vi "GUI.Config Test.vi"(11 "Path Config file":path=path "C:/Trabajo/Test Asic Javi_2021/CONFIG/configuracion_produccion+10mV_CTAV2022A.test") -> (3 "Path out":path)   [LabVIEW 2019]
uses:
  test.test de configuracion gui.ctl
  Test.ctl
  TEST.TEST CONFIG HW.ctl
  Rigol DP832/DP832_Control Channels.ctl
  TEST.TEST CONFIG TEST MATRIZ.ctl
  TEST.TEST CONFIG TEST.ctl
  TEST.TEST RESULT.ctl
  test_result fvasic.ctl
  TEST.TEST EXECUTION TEST.ctl
  TEST.TEST CONFIG VGA.ctl
  TEST.TEST TEST INFO.ctl
  TEST.TEST INFO PC.ctl
  GenPulse_configurar.ctl
  machine estate configs.ctl
  Test_Conjunto Folder/Rigol DP832/DP832_Control Behavior.ctl
panel:
  out "CONFIG GEN temp":T1[](array[typedef]) {"Vasic Theorical" min=1.0 max=1000000.0 step=1.0 format="%#_6pV"; "Frequency" min=0.001 max=333000000.0 step=1000.0 format="%#_6pHz"; "Leading Edge Time" min=1e-09 max=1.0 step=1e-10 format="%#_6ps"; "Trailing Edge Time" min=1e-09 max=1.0 step=1e-10 format="%#_6ps"; "Delay" min=0.0 max=1.0 step=1e-12 format="%#_6ps"; "Trigger Level Sync" items=["ECL", "TTL"]; "Trigger Sync Out" items=["AB"=3, "B"=2, "A"=1, "None"=0]; "Load" min=1.0 max=1000000.0 step=1.0 format="%#_6p"; "DC Offset" min=-10.0 max=10.0 step=0.1 format="%#_6pV"; "Amplitude" min=0.05 max=5.0 step=0.001 format="%#_6pV"; "Width Time" min=1.5e-09 max=1.0 step=1e-10 format="%#_6ps"; "Channel" items=["Channel1"=1, "Channel2"=2]}
  out "Primera llamada":bool=TRUE
  in  "CHECK vga":bool
  in  "VGA":T2={"VALUES VGA"=[], "TIME VGA"={"PULSE WIDTH"=0, "FRECUENCY PULSE"=0.0}} {"TIME VGA"."FRECUENCY PULSE" format="%.3p"; "TIME VGA"."PULSE WIDTH" format="%04x"}
  out "FT_Handle":u32
  in  "Test":T3={"Config HW"={"VISA Rigol DP832"="Rigol_DP832", "Config Rigol DP832"=[{"Channel"=0, "V Limit"=5.5, "I Limit"=0.5, "V Out"=5.0}, {"Channel"=1, "V Limit"=5.5, "I Limit"=0.8, "V Out"=5.0}, {"Channel"=2, "V Limit"=5.5, "I Limit"=0.2, "V Out"=0.0}], "CTA Test#"="CTA013 A", "FT_Handle"=0, "Espera acceso FT"=10, "VISA Tek MDO3104"="Rigol_DP832", "VISA Key 81160A"="Rigol_DP832"}, "Config Test"=[{"Vasic"=2.8, "Global Reset"=FALSE, "Test Register?"=FALSE, "Test ADC?"=FALSE, "Test ADC"={"Repeats ADC"=100, "Max Desviation"=0.1}, "Limits ADC"={"Low"=[1.9, 1.3, 0.65, 0.0, 1.6, 1.4, 1.4, 0.9, 2.1, 0.85, 1.9], "High"=[2.1, 1.5, 0.85, 0.1, 1.4, 1.2, 1.2, 0.7, 1.9, 0.65, 1.7]}, "Test Max PN Min NP?"=FALSE, "Limits Max PN Min NP"={"Max P Upper"=2.177000045776367, "Min P Upper"=1.474, "Max N Upper"=1.475, "Min N Upper"=0.818, "Max P Lower"=1.888, "Min P Lower "=1.321, "Max N Lower"=1.322, "Min N Lower"=0.73}, "Test Rate Scan?"=FALSE, "Vin Rate Scan"=[], "Limits Rate Scan"={"High"=[0.15, 0.242, 0.331, 0.425, 0.512, 0.6, 0.688, 0.774, 0.847, 0.91], "Low"=[0.021, 0.11, 0.189, 0.27, 0.347, 0.421, 0.487, 0.551, 0.601, 0.635]}, "Test Rate Scan Adders?"=FALSE, "Vin Rate Adders"=[], "Limits Rate Scan adders"={"High"=[], "Low"=[]}, "Test offset analog?"=FALSE, "Lim Offset Analog"={"Max Analog"=0.05, "Min Analog"=-0.05}, "Test offset digital?"=FALSE, "Lim offset Dig"={"Max Dig"=0.05}, "Vasic real f.a."=2.8, "IBIAS"=FALSE, "VALUE IBIAS"=63}, {"Vasic"=2.8, "Global Reset"=FALSE, "Test Register?"=FALSE, "Test ADC?"=FALSE, "Test ADC"={"Repeats ADC"=100, "Max Desviation"=0.1}, "Limits ADC"={"Low"=[1.9, 1.3, 0.65, 0.0, 1.6, 1.4, 1.4, 0.9, 2.1, 0.85, 1.9], "High"=[2.1, 1.5, 0.85, 0.1, 1.4, 1.2, 1.2, 0.7, 1.9, 0.65, 1.7]}, "Test Max PN Min NP?"=FALSE, "Limits Max PN Min NP"={"Max P Upper"=2.177000045776367, "Min P Upper"=1.474, "Max N Upper"=1.475, "Min N Upper"=0.818, "Max P Lower"=1.888, "Min P Lower "=1.321, "Max N Lower"=1.322, "Min N Lower"=0.73}, "Test Rate Scan?"=FALSE, "Vin Rate Scan"=[], "Limits Rate Scan"={"High"=[0.15, 0.242, 0.331, 0.425, 0.512, 0.6, 0.688, 0.774, 0.847, 0.91], "Low"=[0.021, 0.11, 0.189, 0.27, 0.347, 0.421, 0.487, 0.551, 0.601, 0.635]}, "Test Rate Scan Adders?"=FALSE, "Vin Rate Adders"=[], "Limits Rate Scan adders"={"High"=[], "Low"=[]}, "Test offset analog?"=FALSE, "Lim Offset Analog"={"Max Analog"=0.05, "Min Analog"=-0.05}, "Test offset digital?"=FALSE, "Lim offset Dig"={"Max Dig"=0.05}, "Vasic real f.a."=2.8, "IBIAS"=FALSE, "VALUE IBIAS"=63}, {"Vasic"=2.8, "Global Reset"=FALSE, "Test Register?"=FALSE, "Test ADC?"=FALSE, "Test ADC"={"Repeats ADC"=100, "Max Desviation"=0.1}, "Limits ADC"={"Low"=[1.9, 1.3, 0.65, 0.0, 1.6, 1.4, 1.4, 0.9, 2.1, 0.85, 1.9], "High"=[2.1, 1.5, 0.85, 0.1, 1.4, 1.2, 1.2, 0.7, 1.9, 0.65, 1.7]}, "Test Max PN Min NP?"=FALSE, "Limits Max PN Min NP"={"Max P Upper"=2.177000045776367, "Min P Upper"=1.474, "Max N Upper"=1.475, "Min N Upper"=0.818, "Max P Lower"=1.888, "Min P Lower "=1.321, "Max N Lower"=1.322, "Min N Lower"=0.73}, "Test Rate Scan?"=FALSE, "Vin Rate Scan"=[], "Limits Rate Scan"={"High"=[0.15, 0.242, 0.331, 0.425, 0.512, 0.6, 0.688, 0.774, 0.847, 0.91], "Low"=[0.021, 0.11, 0.189, 0.27, 0.347, 0.421, 0.487, 0.551, 0.601, 0.635]}, "Test Rate Scan Adders?"=FALSE, "Vin Rate Adders"=[], "Limits Rate Scan adders"={"High"=[], "Low"=[]}, "Test offset analog?"=FALSE, "Lim Offset Analog"={"Max Analog"=0.05, "Min Analog"=-0.05}, "Test offset digital?"=FALSE, "Lim offset Dig"={"Max Dig"=0.05}, "Vasic real f.a."=2.8, "IBIAS"=FALSE, "VALUE IBIAS"=63}, {"Vasic"=2.8, "Global Reset"=FALSE, "Test Register?"=FALSE, "Test ADC?"=FALSE, "Test ADC"={"Repeats ADC"=100, "Max Desviation"=0.1}, "Limits ADC"={"Low"=[1.9, 1.3, 0.65, 0.0, 1.6, 1.4, 1.4, 0.9, 2.1, 0.85, 1.9], "High"=[2.1, 1.5, 0.85, 0.1, 1.4, 1.2, 1.2, 0.7, 1.9, 0.65, 1.7]}, "Test Max PN Min NP?"=FALSE, "Limits Max PN Min NP"={"Max P Upper"=2.177000045776367, "Min P Upper"=1.474, "Max N Upper"=1.475, "Min N Upper"=0.818, "Max P Lower"=1.888, "Min P Lower "=1.321, "Max N Lower"=1.322, "Min N Lower"=0.73}, "Test Rate Scan?"=FALSE, "Vin Rate Scan"=[], "Limits Rate Scan"={"High"=[0.15, 0.242, 0.331, 0.425, 0.512, 0.6, 0.688, 0.774, 0.847, 0.91], "Low"=[0.021, 0.11, 0.189, 0.27, 0.347, 0.421, 0.487, 0.551, 0.601, 0.635]}, "Test Rate Scan Adders?"=FALSE, "Vin Rate Adders"=[], "Limits Rate Scan adders"={"High"=[], "Low"=[]}, "Test offset analog?"=FALSE, "Lim Offset Analog"={"Max Analog"=0.05, "Min Analog"=-0.05}, "Test offset digital?"=FALSE, "Lim offset Dig"={"Max Dig"=0.05}, "Vasic real f.a."=2.8, "IBIAS"=FALSE, "VALUE IBIAS"=63}], "Result"=[], "Execucion Test"={"Vasic Actual"=0}, "Config VGA"={"Theoretical Voltage"=[0.1, 0.2, 0.3, 0.4, 0.5, 0.6, 0.7, 0.8, 0.9, 1.0], "Real Voltage"=[0.10285, 0.20714, 0.29957, 0.40485, 0.49571, 0.60685, 0.69771, 0.80114, 0.89714, 0.99885], "Pulse Width"=57344, "Frecuency Pulse"=1000000.0, "VGA Gain"=[9, 16, 24, 34, 43, 52, 61, 72, 81, 93]}, "Test Info"={"Asic"="", "Operator"="", "Place"="", "Time start"=timestamp(0 s since 1904-01-01), "Time stop"=timestamp(0 s since 1904-01-01)}, "Info machine"={"SO"="", "SO Name"="", "SO Ver"="", "SO Build"="", "CPU"="", "APP"="", "APP YEAR"="", "APP ver"="", "APP User"="", "APP Serail"="", "MAC"=[], "PC NAME"=[], "PC IP"=[], "BIOS MANU"="", "BIOS NAME"="", "BIOS SERIAL"="", "BOARD MANU"="", "BOARD NAME"="", "BOARD SERIAL"="", "Driver Version"="", "Library Version"="", "FPGA Ver"=0, "ID CTA board"=0, "LAST BOOT"="", "LABVIEW Ver"=0}, "Partial Report"="", "CONFIG GEN"=[]} {"CONFIG GEN"."Vasic Theorical" min=1.0 max=1000000.0 step=1.0 format="%#_6pV"; "CONFIG GEN"."Frequency" min=0.001 max=333000000.0 step=1000.0 format="%#_6pHz"; "CONFIG GEN"."Leading Edge Time" min=1e-09 max=1.0 step=1e-10 format="%#_6ps"; "CONFIG GEN"."Trailing Edge Time" min=1e-09 max=1.0 step=1e-10 format="%#_6ps"; "CONFIG GEN"."Delay" min=0.0 max=1.0 step=1e-12 format="%#_6ps"; "CONFIG GEN"."Trigger Level Sync" items=["ECL", "TTL"]; "CONFIG GEN"."Trigger Sync Out" items=["AB"=3, "B"=2, "A"=1, "None"=0]; "CONFIG GEN"."Load" min=1.0 max=1000000.0 step=1.0 format="%#_6p"; "CONFIG GEN"."DC Offset" min=-10.0 max=10.0 step=0.1 format="%#_6pV"; "CONFIG GEN"."Amplitude" min=0.05 max=5.0 step=0.001 format="%#_6pV"; "CONFIG GEN"."Width Time" min=1.5e-09 max=1.0 step=1e-10 format="%#_6ps"; "CONFIG GEN"."Channel" items=["Channel1"=1, "Channel2"=2]; "Config VGA"."Theoretical Voltage" format="%1.4f"; "Config VGA"."VGA Gain" format="%02x"; "Config VGA"."Frecuency Pulse" format="%0_2p"; "Config VGA"."Pulse Width" format="%04x"; "Config VGA"."Real Voltage" format="%1.5f"; "Config Test"."VALUE IBIAS" max=63 step=1; "Config Test"."Vasic real f.a." min=2.8 max=3.8 step=0.01 format="%.2g"; "Config Test"."Limits Rate Scan adders"."Low" format="%1.3f"; "Config Test"."Limits Rate Scan adders"."High" format="%1.3f"; "Config Test"."Limits ADC"."High" format="%1.4f"; "Config Test"."Limits ADC"."Low" format="%1.3f"; "Config Test"."Lim offset Dig"."Max Dig" format="%.3g"; "Config Test"."Lim Offset Analog"."Min Analog" format="%.3g"; "Config Test"."Lim Offset Analog"."Max Analog" format="%.3g"; "Config Test"."Limits Rate Scan"."Low" format="%1.4f"; "Config Test"."Limits Rate Scan"."High" format="%1.3f"; "Config Test"."Limits Max PN Min NP"."Min P Upper" format="%.3g"; "Config Test"."Limits Max PN Min NP"."Min P Lower" format="%.3g"; "Config Test"."Limits Max PN Min NP"."Max N Lower" format="%.3g"; "Config Test"."Limits Max PN Min NP"."Max N Upper" format="%.3g"; "Config Test"."Limits Max PN Min NP"."Min N Lower" format="%.3g"; "Config Test"."Limits Max PN Min NP"."Min N Upper" format="%.3g"; "Config Test"."Limits Max PN Min NP"."Max P Upper" format="%.3g"; "Config Test"."Limits Max PN Min NP"."Max P Lower" format="%.3g"; "Config Test"."Vasic" min=2.8 max=3.8 step=0.01 format="%.2g"; "Config HW"."Config Rigol DP832"."Channel" items=["+30V Channel 1", "+30V Channel 2", "+5V Channel 3"]; "Config HW"."Config Rigol DP832"."V Limit" format="%.1g"; "Config HW"."Config Rigol DP832"."I Limit" format="%.1g"; "Config HW"."Config Rigol DP832"."V Out" format="%.1g"; "Result"."Test Registros"."Read W/R" format="%04x"; "Result"."Test Registros"."Pattern W/R" format="%04x"; "Result"."Test Registros"."Read Default" format="%04x"; "Result"."Test Registros"."Pattern Default" format="%04x"}
  in  "visualize":enum32{"Page 1", "Page 2"}(tab)
  in  "Change value Gen":bool
  in  "VISA Oscilloscope Tek MDO3104":refnum<visa-resource-name>
  in  "VISA Generator Key 81160A":refnum<visa-resource-name>
  in  "Elemensts":i32(listbox)=-1
  in  "vga test":T14={"FRECUENCY PULSE"=-0.05, "PULSE WIDTH"=0, "CODE GAIN TEST"=0} {"CODE GAIN TEST" max=127 step=1; "PULSE WIDTH" format="%04x"; "FRECUENCY PULSE" format="%.3p"}
  in  "CTA Board":string(combo)
  in  "CHECK cta":bool
  in  "CHECK POWER":bool
  in  "Config Rigol DP832":T15(array[cluster]) {"Channel" items=["+30V Channel 1", "+30V Channel 2", "+5V Channel 3"]; "V Limit" min=0.0 max=6.0 step=0.1 format="%.1g"; "I Limit" min=0.0 max=1.0 step=0.1 format="%.1g"; "V Out" min=0.0 max=6.0 step=0.01 format="%.2g"}
  in  "copy to new":bool
  in  "new":bool
  in  "delete":bool
  in  "Valores":T16[](array[typedef]) {"VALUE IBIAS" max=63 step=1; "V SUPPLY ASIC REAL" min=2.5 max=3.6 step=0.01 format="%.2g"; "VOLTAGE SUPPLY ASIC" min=2.5 max=3.5 step=0.05 format="%.2g"; "LIMITS OFFSET DIGITAL"."MAXIMUM" format="%.3g"; "LIMITS OFFSET ANALOG"."MINIMUM" format="%.3g"; "LIMITS OFFSET ANALOG"."MAXIMUM" format="%.3g"; "SETUP ADC"."MAX DESVIATION ADC" format="%.3g"}
  in  "default":bool
  in  "Load config":bool
  in  "save config":bool
  in  "QUIT":bool
  in  "VISA Rigol DP832":refnum<visa-resource-name>
  out "Values Gen":string[][](table)
  out "Cambios":bool
  # "Modo 2\nModo 3\nModo 4\nModo 2\nModo 3\nModo 4"
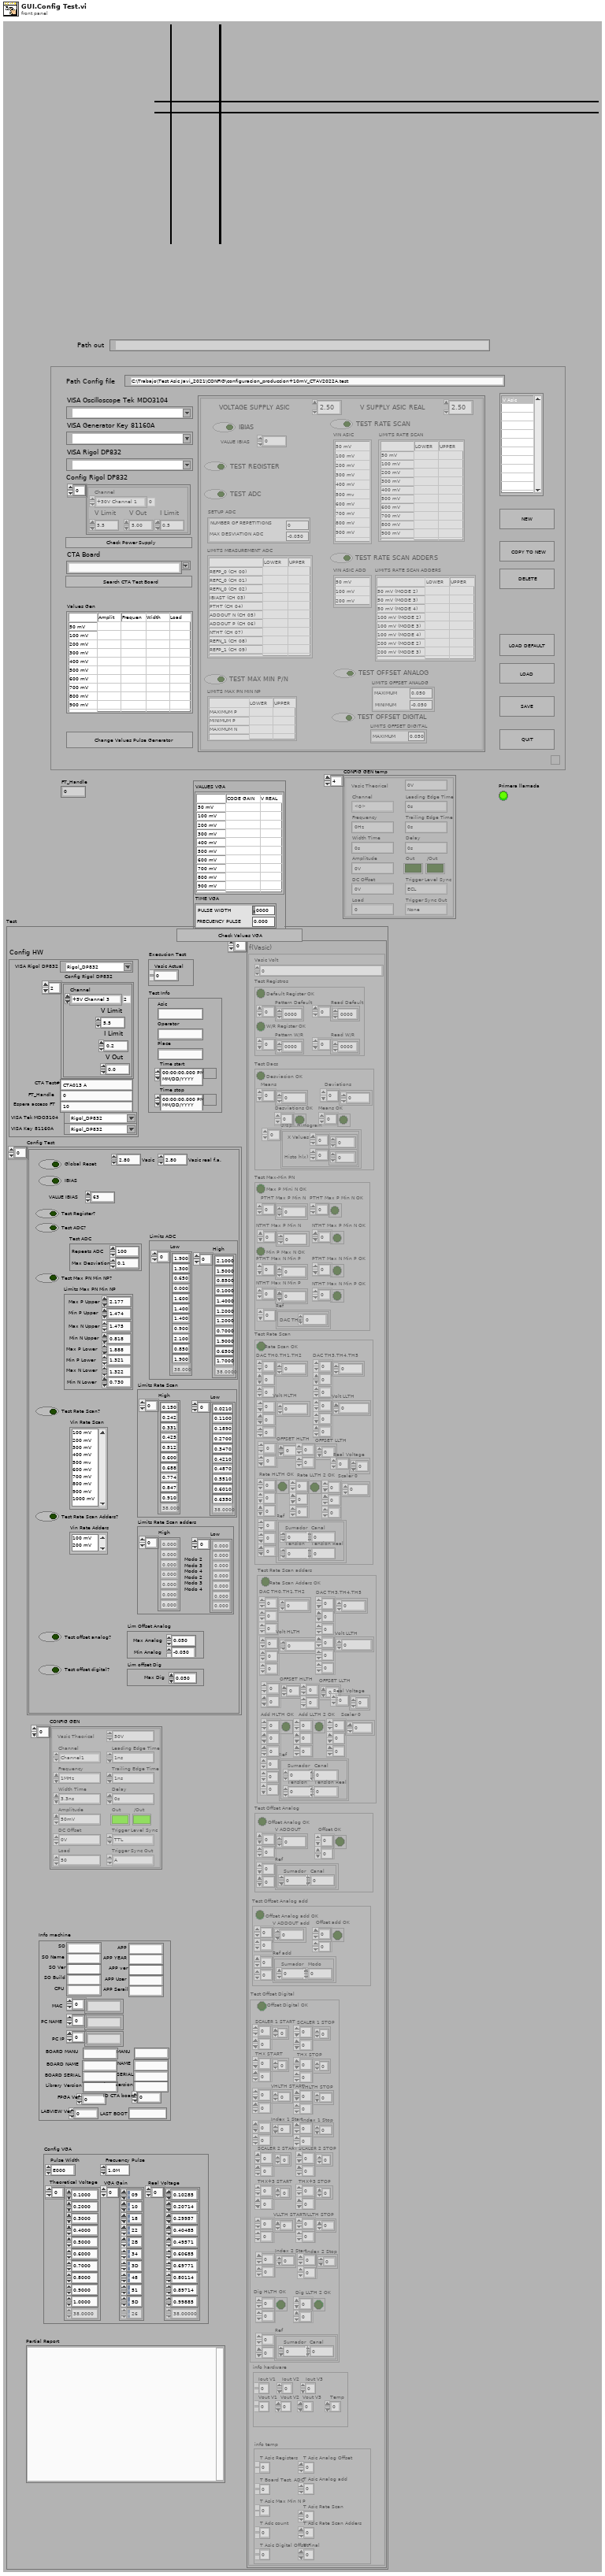
[diagram p1: front panel]
types:
  T1 = typedef "GenPulse_configurar.ctl" = cluster{"Channel":u16, "Frequency":dbl, "Width Time":dbl, "Amplitude":dbl, "DC Offset":dbl, "Load":dbl, "Leading Edge Time":dbl, "Trailing Edge Time":dbl, "Delay":dbl, "Out":bool, "/Out":bool, "Trigger Level Sync":u16, "Trigger Sync Out":u16, "Vasic Theorical":dbl}
  T2 = cluster{"VALUES VGA":string[][], "TIME VGA":cluster{"PULSE WIDTH":u16, "FRECUENCY PULSE":dbl}}
  T3 = typedef "Test.ctl" = cluster{"Config HW":T4, "Config Test":T6, "Result":T8, "Execucion Test":T10, "Config VGA":T11, "Test Info":T12, "Info machine":T13, "Partial Report":string, "CONFIG GEN":T1[]}
  T4 = typedef "TEST.TEST CONFIG HW.ctl" = cluster{"VISA Rigol DP832":refnum<visa-resource-name>, "Config Rigol DP832":cluster{"Channel":T5, "V Limit":dbl, "I Limit":dbl, "V Out":dbl}[], "CTA Test#":string, "FT_Handle":u32, "Espera acceso FT":u32, "VISA Tek MDO3104":refnum<visa-resource-name>, "VISA Key 81160A":refnum<visa-resource-name>}
  T5 = typedef "DP832_Control Channels.ctl" = i32
  T6 = typedef "TEST.TEST CONFIG TEST MATRIZ.ctl" = T7[]
  T7 = typedef "TEST.TEST CONFIG TEST.ctl" = cluster{"Vasic":dbl, "Global Reset":bool, "Test Register?":bool, "Test ADC?":bool, "Test ADC":cluster{"Repeats ADC":i32, "Max Desviation":dbl}, "Limits ADC":cluster{"Low":dbl[], "High":dbl[]}, "Test Max PN Min NP?":bool, "Limits Max PN Min NP":cluster{"Max P Upper":dbl, "Min P Upper":dbl, "Max N Upper":dbl, "Min N Upper":dbl, "Max P Lower":dbl, "Min P Lower ":dbl, "Max N Lower":dbl, "Min N Lower":dbl}, "Test Rate Scan?":bool, "Vin Rate Scan":i32[], "Limits Rate Scan":cluster{"High":dbl[], "Low":dbl[]}, "Test Rate Scan Adders?":bool, "Vin Rate Adders":i32[], "Limits Rate Scan adders":cluster{"High":dbl[], "Low":dbl[]}, "Test offset analog?":bool, "Lim Offset Analog":cluster{"Max Analog":dbl, "Min Analog":dbl}, "Test offset digital?":bool, "Lim offset Dig":cluster{"Max Dig":dbl}, "Vasic real f.a.":dbl, "IBIAS":bool, "VALUE IBIAS":u8}
  T8 = typedef "TEST.TEST RESULT.ctl" = T9[]
  T9 = typedef "test_result fvasic.ctl" = cluster{"Vasic Volt":i32, "Test Registros":cluster{"Default Register OK":bool, "Pattern Default":u16[], "Read Default":u16[], "W/R Register OK":bool, "Pattern W/R":u16[], "Read W/R":u16[]}, "Test Dacs":cluster{"Desviacion OK":bool, "Means":dbl[], "Deviations":dbl[], "Desviations OK":bool[], "Means OK":bool[], "Graph Histogram":cluster{"X Values":dbl[], "Histo h(x)":i32[]}[]}, "Test Max-Min PN":cluster{"Max P Mini N OK":bool, "PTHT Max P Min N":dbl[], "PTHT Max P Min N OK":bool[], "NTHT Max P Min N":dbl[], "NTHT Max P Min N OK":bool[], "Min P Max N OK":bool, "PTHT Max N Min P":dbl[], "PTHT Max N Min P OK":bool[], "NTHT Max N Min P":dbl[], "NTHT Max N Min P OK":bool[], "Ref":cluster{"DAC THx":u8}[]}, "Test Rate Scan":cluster{"Rate Scan OK":bool, "DAC TH0,TH1,TH2":u16[][][], "Volt HLTH":dbl[][][], "Rate HLTH OK":bool[][][], "DAC TH3,TH4,TH5":u16[][][], "Volt LLTH":dbl[][][], "Rate LLTH 2 OK":bool[][][], "Scaler 0":u16[][][], "Ref":cluster{"Sumador":u8, "Canal":u8, "Tension":u8, "Tension Real":dbl}[][][], "OFFSET HLTH":dbl[][], "OFFSET LLTH":dbl[][], "Real Voltage":dbl[]}, "Test Rate Scan adders":cluster{"Rate Scan Adders OK":bool, "DAC TH0,TH1,TH2":u16[][][], "Volt HLTH":dbl[][][], "Add HLTH OK":bool[][][], "DAC TH3,TH4,TH5":u16[][][], "Volt LLTH":dbl[][][], "Add LLTH 2 OK":bool[][][], "Scaler 0":u16[][][], "Ref":cluster{"Sumador":u8, "Canal":u8, "Tension":u8, "Tension Real":dbl}[][][], "OFFSET HLTH":dbl[][], "OFFSET LLTH":dbl[][], "Real Voltage":dbl[]}, "Test Offset Analog":cluster{"Offset Analog OK":bool, "V ADDOUT":dbl[][], "Offset OK":bool[][], "Ref":cluster{"Sumador":u8, "Canal":u8}[][]}, "Test Offset Digital":cluster{"Offset Digital OK":bool, "SCALER 1 START":u16[][], "SCALER 1 STOP":u16[][], "THX START":u16[][], "THX STOP":u16[][], "VHLTH START":dbl[][], "VHLTH STOP":dbl[][], "Index 1 Start":i32[][], "index 1 Stop":i32[][], "SCALER 2 START":u16[][], "SCALER 2 STOP":u16[][], "THX+3 START":u16[][], "THX+3 STOP":u16[][], "VLLTH START":dbl[][], "VLLTH STOP":dbl[][], "Index 2 Start":i32[][], "index 2 Stop":i32[][], "Dig HLTH OK":bool[][], "Dig LLTH 2 OK":bool[][], "Ref":cluster{"Sumador":u8, "Canal":u8}[][]}, "info hardware":cluster{"Iout V1":dbl, "Iout V2":dbl, "Iout V3":dbl, "Vout V1":dbl, "Vout V2":dbl, "Vout V3":dbl, "Temp":dbl}, "Test Offset Analog add":cluster{"Offset Analog add OK":bool, "V ADDOUT add":dbl[][], "Offset add OK":bool[][], "Ref add":cluster{"Sumador":u8, "Modo":u8}[][]}, "info temp":cluster{"T Asic Registers":dbl, "T Board Test. ADC":dbl, "T Asic Max Min N P":dbl, "T Adc count":dbl, "T Asic Digital Offset":dbl, "T Asic Analog Offset":dbl, "T Asic Analog add":dbl, "T Asic Rate Scan":dbl, "T Asic Rate Scan Adders":dbl, "T Final":dbl}}
  T10 = typedef "TEST.TEST EXECUTION TEST.ctl" = cluster{"Vasic Actual":i32}
  T11 = typedef "TEST.TEST CONFIG VGA.ctl" = cluster{"Theoretical Voltage":dbl[], "Real Voltage":dbl[], "Pulse Width":u16, "Frecuency Pulse":dbl, "VGA Gain":u8[]}
  T12 = typedef "TEST.TEST TEST INFO.ctl" = cluster{"Asic":string, "Operator":string, "Place":string, "Time start":timestamp, "Time stop":timestamp}
  T13 = typedef "TEST.TEST INFO PC.ctl" = cluster{"SO":string, "SO Name":string, "SO Ver":string, "SO Build":string, "CPU":string, "APP":string, "APP YEAR":string, "APP ver":string, "APP User":string, "APP Serail":string, "MAC":string[], "PC NAME":string[], "PC IP":string[], "BIOS MANU":string, "BIOS NAME":string, "BIOS SERIAL":string, "BOARD MANU":string, "BOARD NAME":string, "BOARD SERIAL":string, "Driver Version":string, "Library Version":string, "FPGA Ver":u8, "ID CTA board":u64, "LAST BOOT":string, "LABVIEW Ver":u32}
  T14 = cluster{"FRECUENCY PULSE":dbl, "PULSE WIDTH":u16, "CODE GAIN TEST":u8}
  T15 = cluster{"Channel":T5, "V Limit":dbl, "I Limit":dbl, "V Out":dbl}[]
  T16 = typedef "test.test de configuracion gui.ctl" = cluster{"VOLTAGE SUPPLY ASIC":dbl, "GLOBAL RESET":bool, "TEST REGISTER":bool, "TEST ADC":bool, "SETUP ADC":cluster{"NUMBER OF REPETITIONS":i32, "MAX DESVIATION ADC":dbl}, "LIMITS MEASUREMENT ADC":string[][], "TEST MAX MIN P/N":bool, "LIMITS MAX PN MIN NP":string[][], "TEST RATE SCAN":bool, "VIN ASIC":i32[], "LIMITS RATE SCAN":string[][], "TEST RATE SCAN ADDERS":bool, "VIN ASIC ADD":i32[], "LIMITS RATE SCAN ADDERS":string[][], "TEST OFFSET ANALOG":bool, "LIMITS OFFSET ANALOG":cluster{"MAXIMUM":dbl, "MINIMUM":dbl}, "TEST OFFSET DIGITAL":bool, "LIMITS OFFSET DIGITAL":cluster{"MAXIMUM":dbl}, "V SUPPLY ASIC REAL":dbl, "VALUE IBIAS":u8, "IBIAS":bool}
  T17 = typedef "machine estate configs.ctl" = enum16{"Default values", "Init", "load init file", "wait", "Load File", "Refresh", "quit", "Save File", "Save In Config", "Valores>Test", "Test>View", "quit save"}
  T18 = cluster{"Config HW":T4, "Config Test":T6, "Config VGA":T11, "CONFIG GEN":T1[]}
  T19 = enum8{"Enabled", "Disabled", "Disabled and Grayed Out"}
  T20 = cluster{"Left Button Key Shortcut":cluster{"Control":bool, "Shift":bool, "Key":string}, "Center Button Key Shortcut":cluster{"Control":bool, "Shift":bool, "Key":string}, "Right Button Key Shortcut":cluster{"Control":bool, "Shift":bool, "Key":string}}
  T21 = cluster{"CTA Test#":string, "CTA Test#":string}[]
  T22 = typedef "DP832_Control Behavior.ctl" = u16
  T23 = cluster{"Device Index":u32, "FT_FLAGS_OPENED":bool, "FT_FLAGS_HISPEED":bool, "Type":u32, "VID":u32, "PID":u32, "LocID":i32, "Serial Number":string, "Description":string, "FT_Handle":u32}[]
  T24 = cluster{"Device Index":u32, "FT_FLAGS_OPENED":bool, "FT_FLAGS_HISPEED":bool, "Type":u32, "VID":u32, "PID":u32, "LocID":i32, "Serial Number":string, "Description":string, "FT_Handle":u32}
  T25 = cluster{"Serial Number":string, "Serial Number":string}
  T26 = cluster{"Vsupply asic":dbl, "Global Reset":bool, "Test Register??":bool, "Test ADC??":bool, "Test ADC set":cluster{"Repeats ADC":i32, "Max Desviation":dbl}, "High ADC means":dbl[], "Low ADC means":dbl[], "Test MAX/MIN??":bool, "Limits Max PN Min NP":cluster{"Max P Lower":dbl, "Min P Lower ":dbl, "Max N Lower":dbl, "Min N Lower":dbl, "Max P Upper":dbl, "Min P Upper":dbl, "Min N Upper":dbl, "Max N Upper":dbl}, "Test rate scan":bool, "Vin Rate Scan":i32[], "High rate scan":dbl[], "Low rate scan":dbl[], "Test rate scan adders??":bool, "Vin Rate Adders":i32[], "High rate scan add":dbl[], "Low rate scan add":dbl[], "Test offset analog??":bool, "Lim Offset Analog":cluster{"Max Analog":dbl, "Min Analog":dbl}, "Test offset digital??":bool, "Lim offset Dig":cluster{"Max Dig":dbl}, "Vsupply asic real":dbl, "IBIAS":bool, "VALUE IBIAS":u8}[]
  T27 = cluster{"Vsupply asic":dbl, "Global Reset":bool, "Test Register??":bool, "Test ADC??":bool, "Test ADC set":cluster{"Repeats ADC":i32, "Max Desviation":dbl}, "High ADC means":dbl[], "Low ADC means":dbl[], "Test MAX/MIN??":bool, "Limits Max PN Min NP":cluster{"Max P Lower":dbl, "Min P Lower ":dbl, "Max N Lower":dbl, "Min N Lower":dbl, "Max P Upper":dbl, "Min P Upper":dbl, "Min N Upper":dbl, "Max N Upper":dbl}, "Test rate scan":bool, "Vin Rate Scan":i32[], "High rate scan":dbl[], "Low rate scan":dbl[], "Test rate scan adders??":bool, "Vin Rate Adders":i32[], "High rate scan add":dbl[], "Low rate scan add":dbl[], "Test offset analog??":bool, "Lim Offset Analog":cluster{"Max Analog":dbl, "Min Analog":dbl}, "Test offset digital??":bool, "Lim offset Dig":cluster{"Max Dig":dbl}, "Vsupply asic real":dbl, "IBIAS":bool, "VALUE IBIAS":u8}
  T28 = enum16{"Left Button", "Center Button", "Right Button", "Window Close"}
  T29 = cluster{"VISA Rigol DP832":refnum<visa-resource-name>, "CTA Test#":string, "VISA Tek MDO3104":refnum<visa-resource-name>, "VISA Key 81160a":refnum<visa-resource-name>}
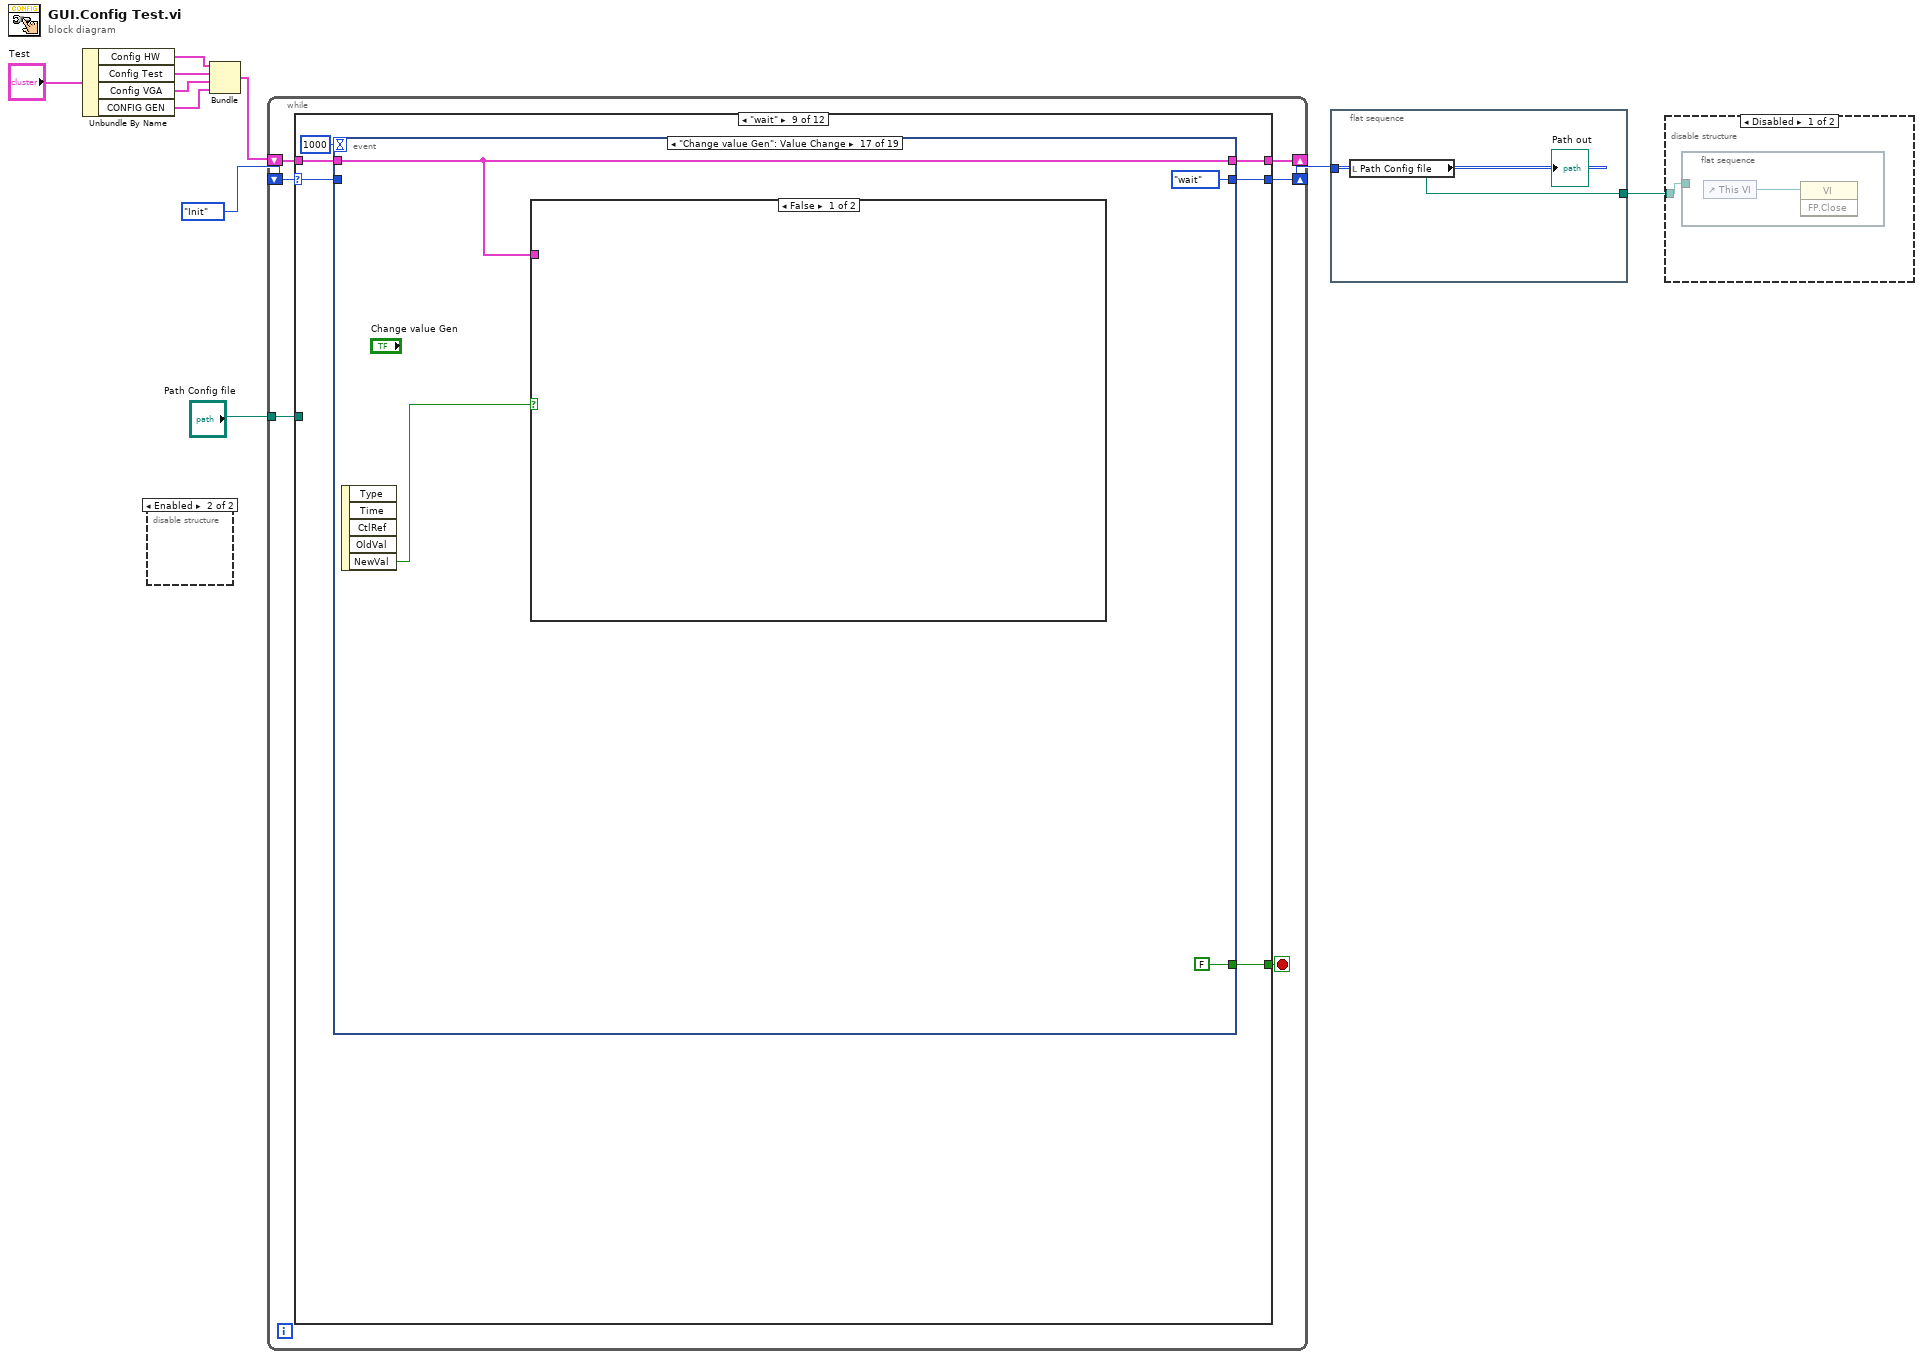
[diagram p0: block diagram]
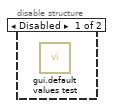
[diagram p3: hidden frame]
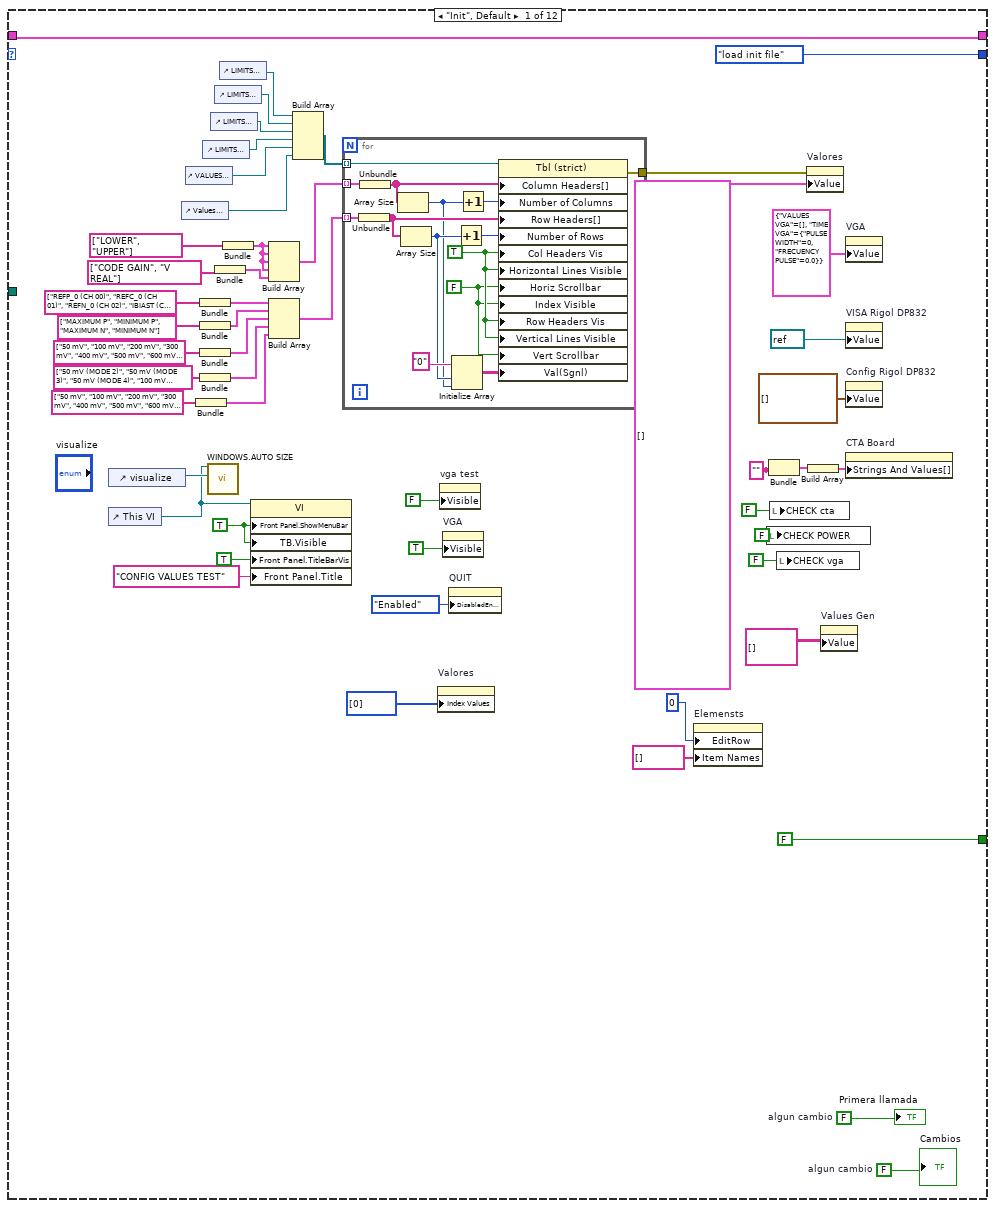
[diagram p4: hidden frame]
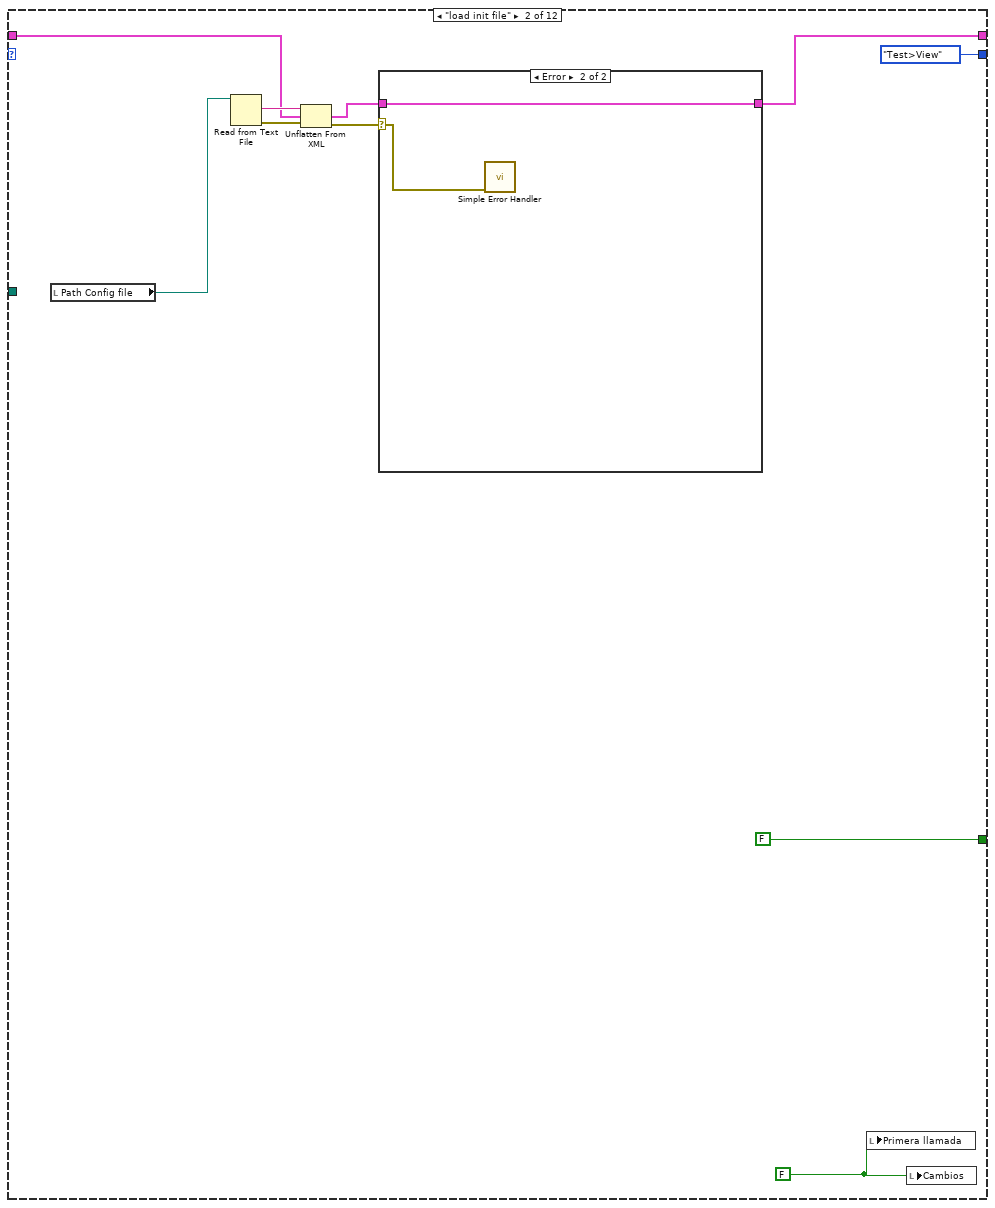
[diagram p5: hidden frame]
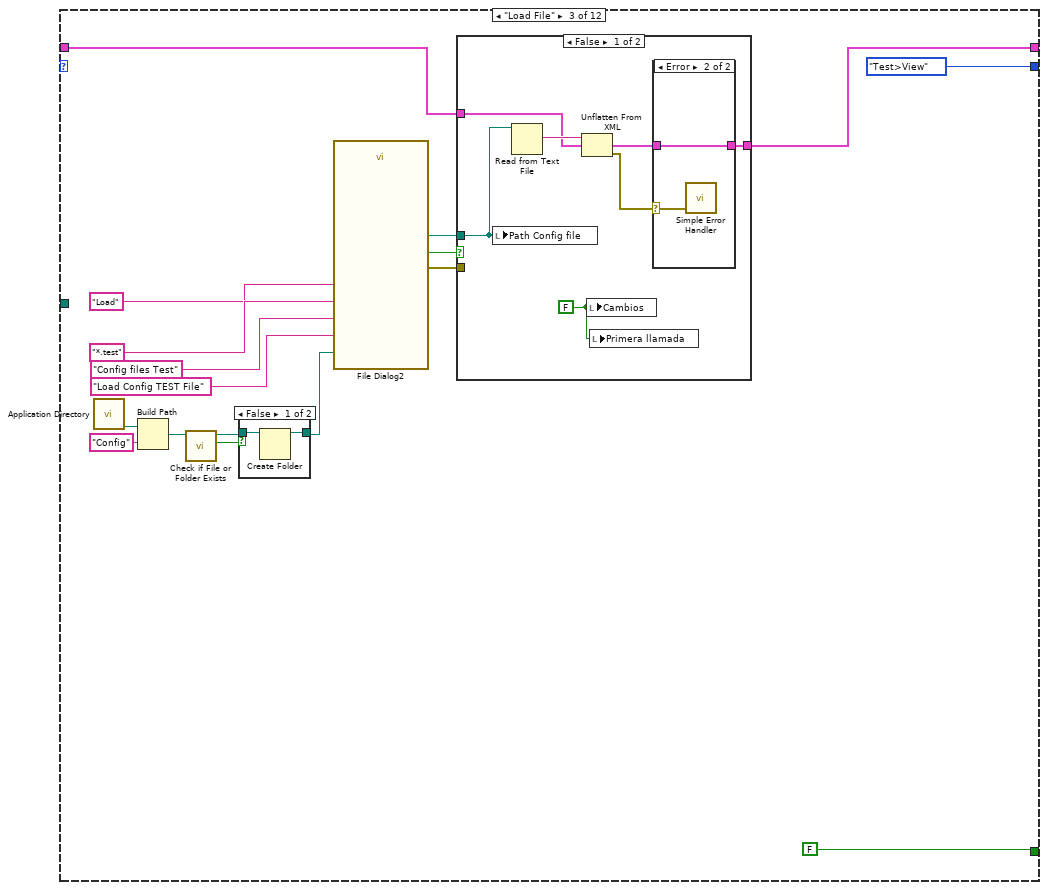
[diagram p7: hidden frame]
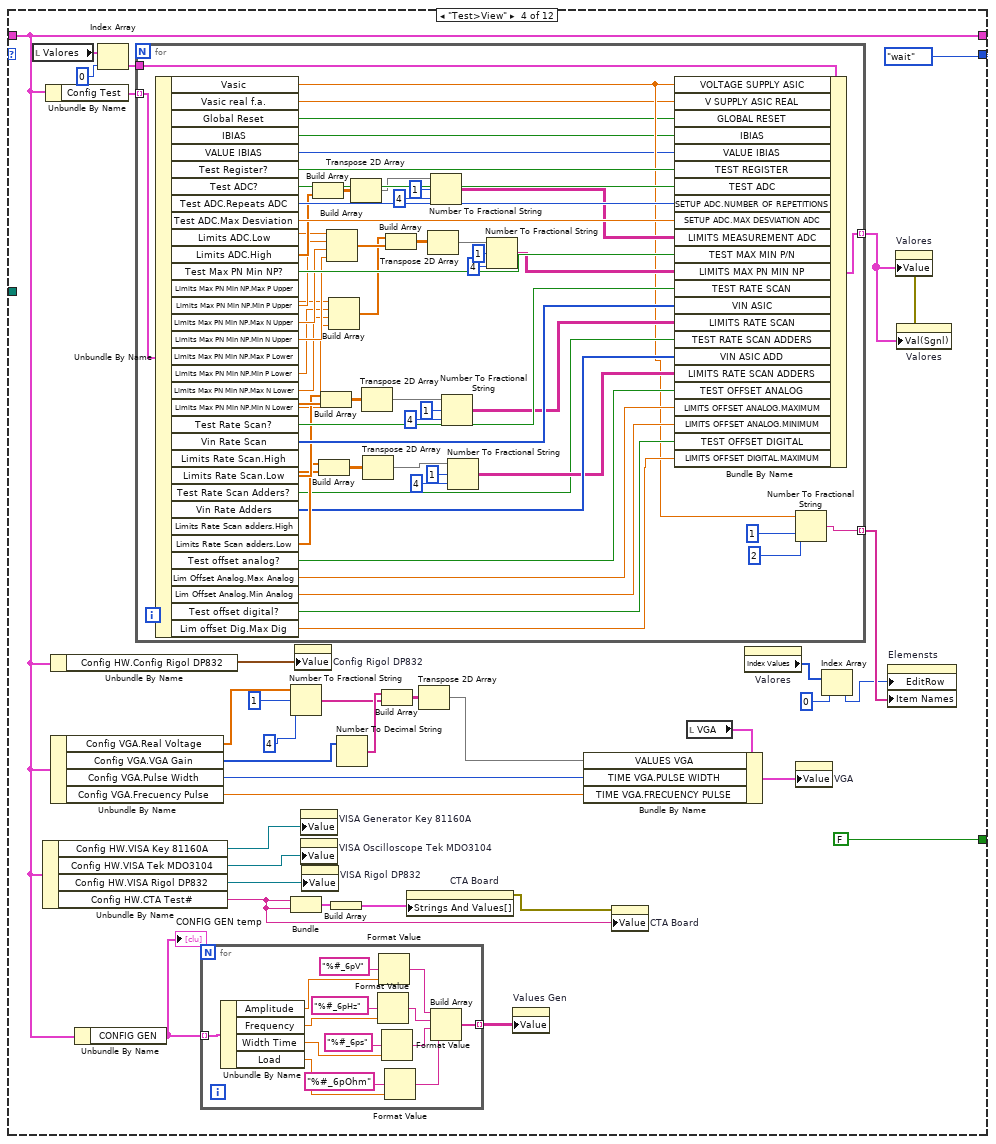
[diagram p11: hidden frame]
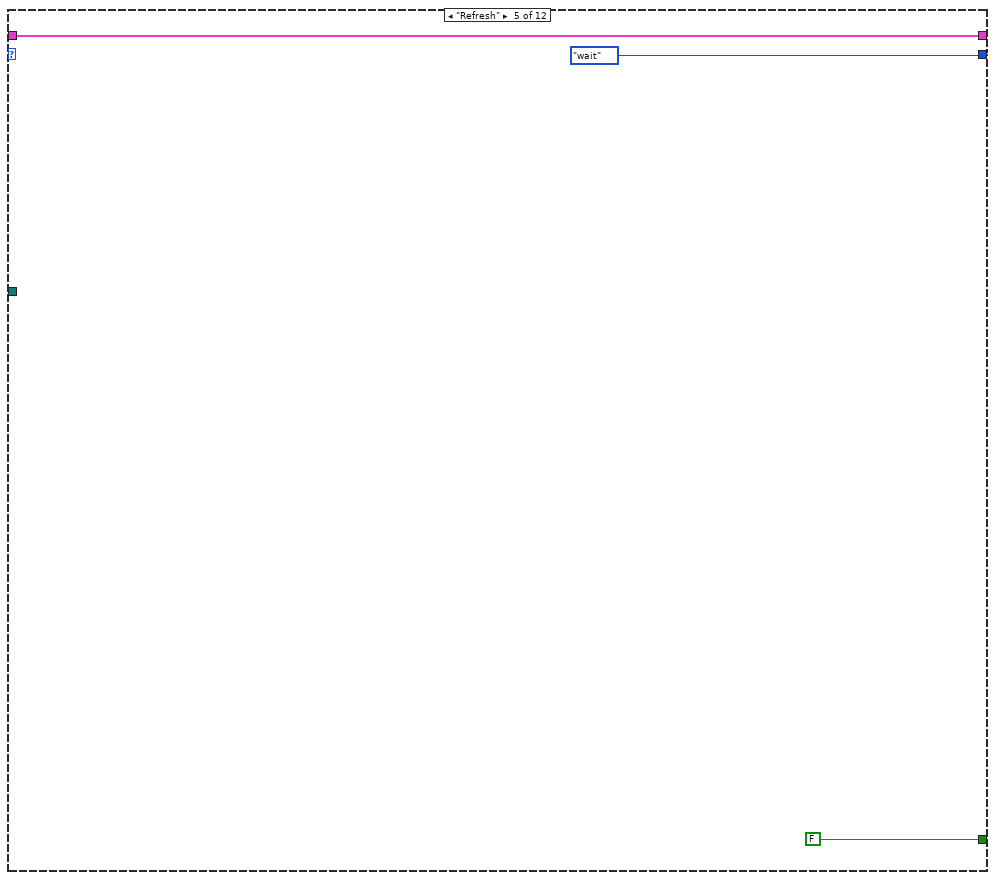
[diagram p12: hidden frame]
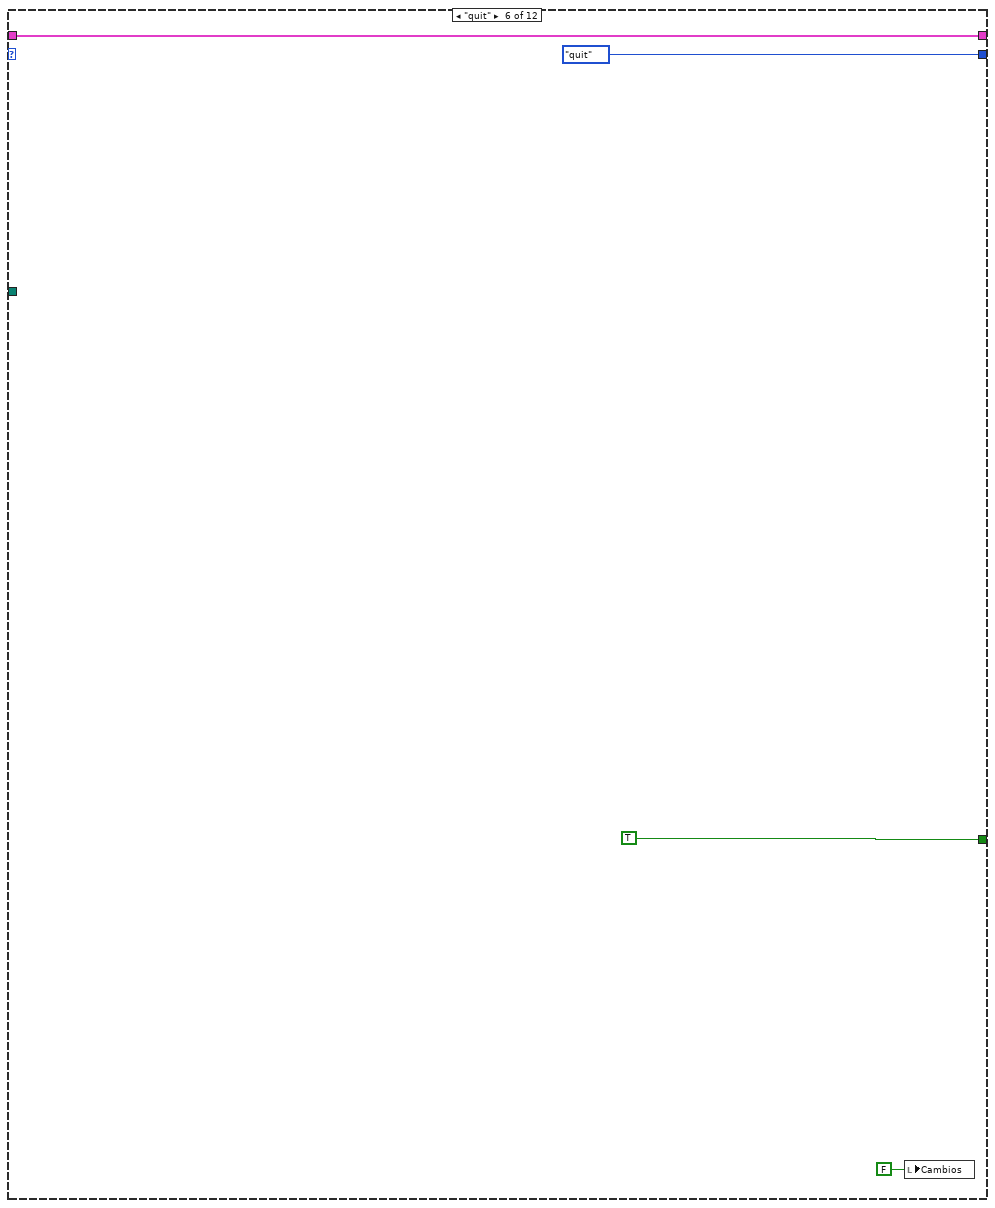
[diagram p13: hidden frame]
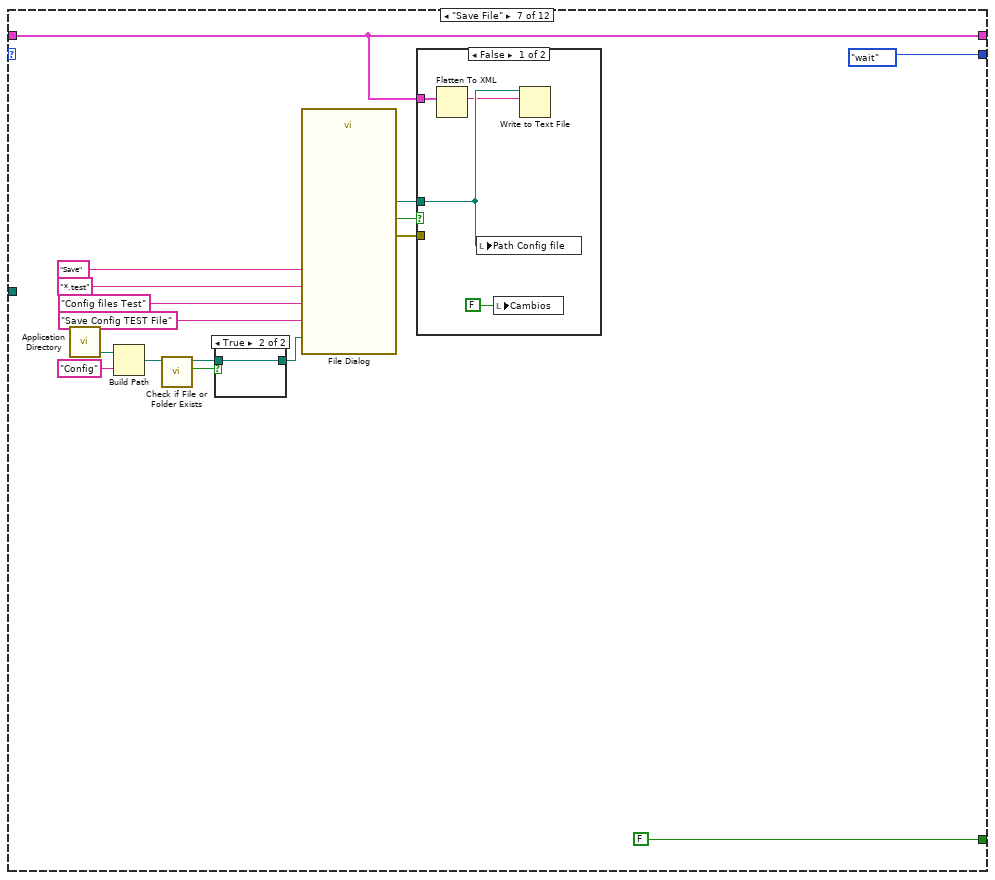
[diagram p14: hidden frame]
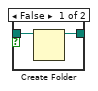
[diagram p16: hidden frame]
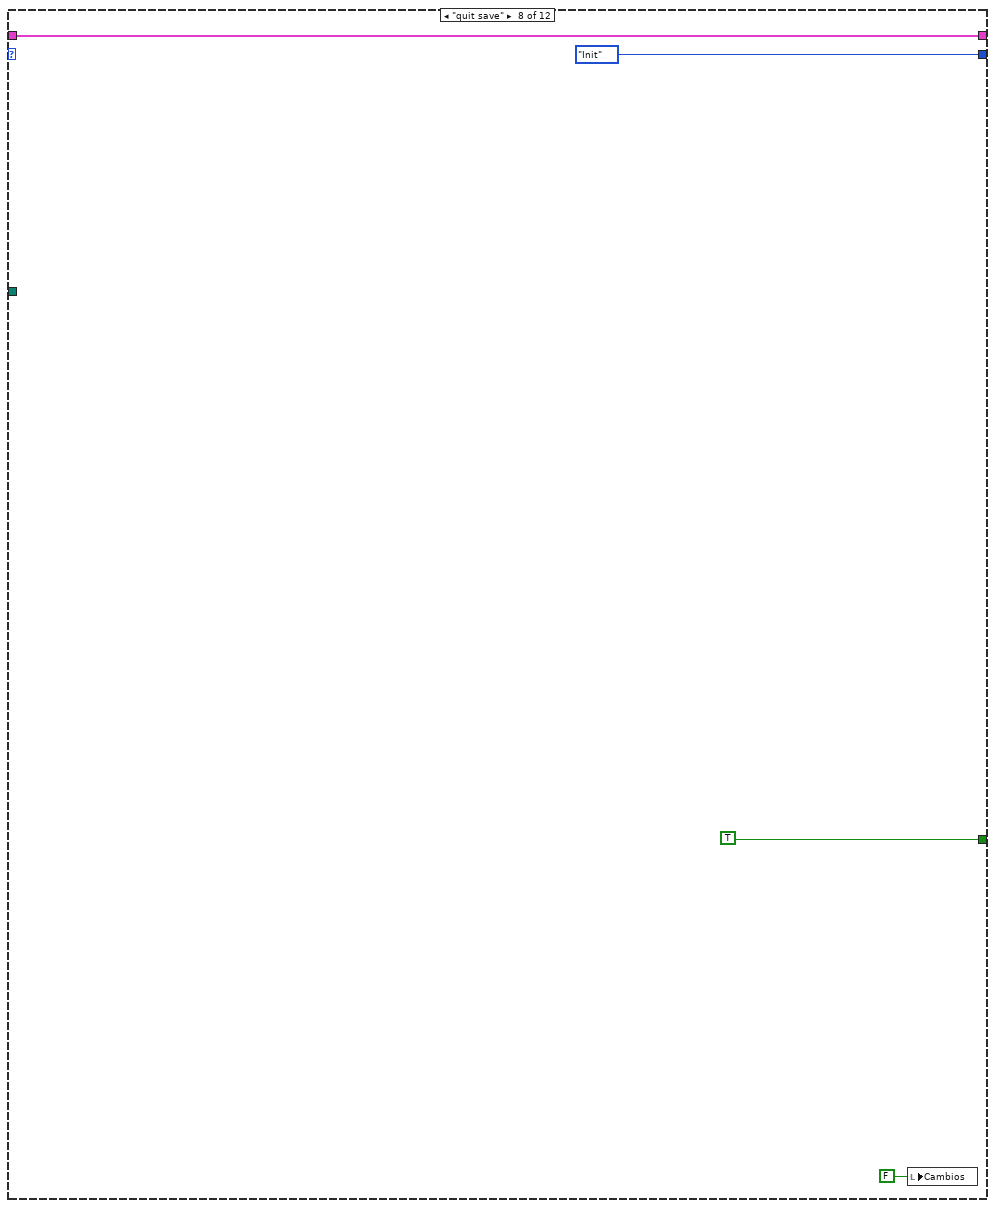
[diagram p17: hidden frame]
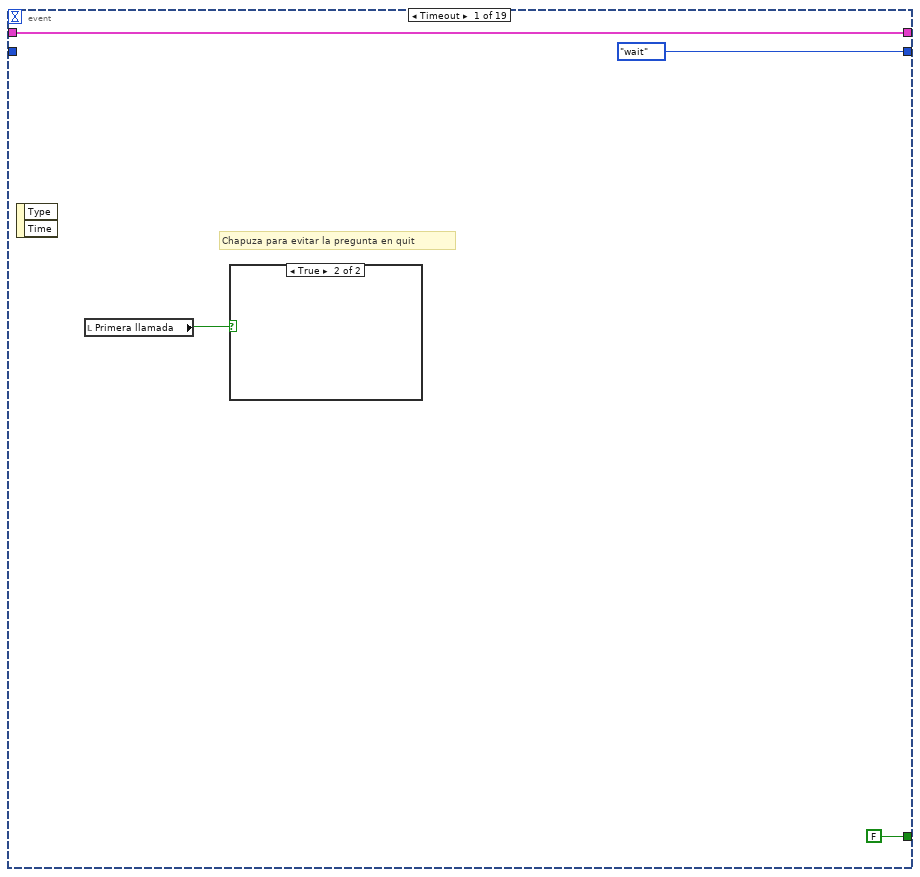
[diagram p18: hidden frame]
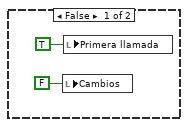
[diagram p19: hidden frame]
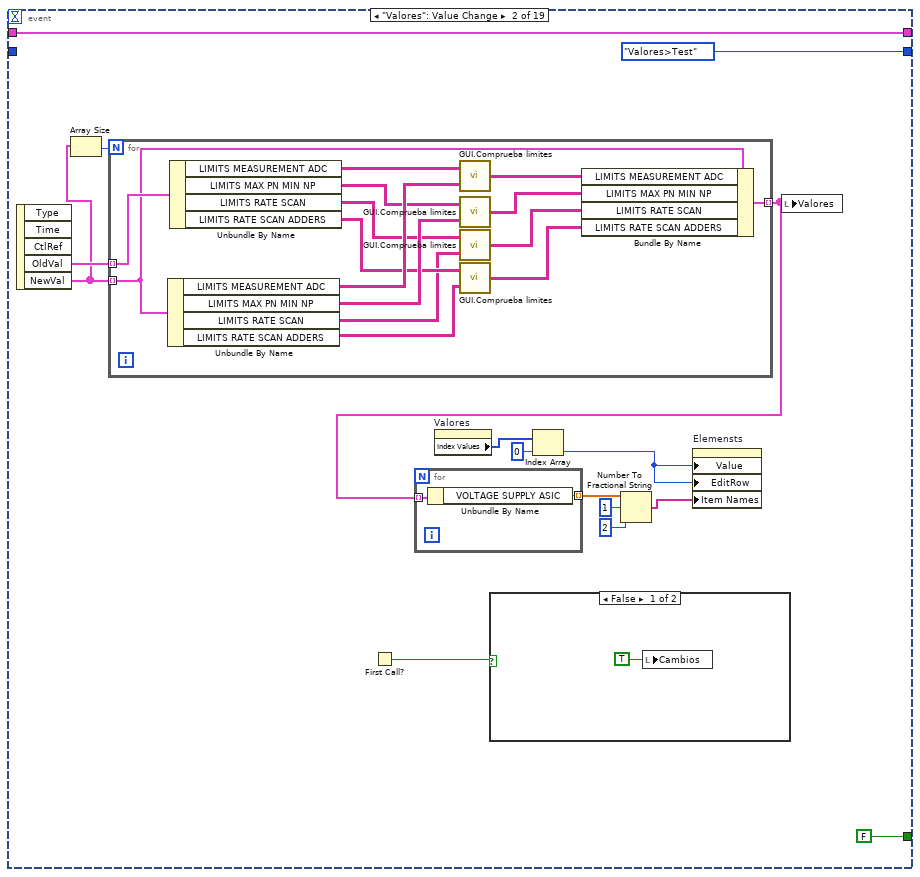
[diagram p20: hidden frame]
diagram:
  n1 = Unbundle By Name("Test") -> ("Config HW"=w5:T4, "Config Test"=w6:T6, "Config VGA"=w7:T11, "CONFIG GEN"=w1:T1[])
  n2 = disable-structure shown="Enabled" {
    frame Disabled {
      n3 = call "gui.default values test.vi"() -> ()  [unwired: 7 in, 5 out]
    }
    frame Enabled {
    }
  }
  n4 = Bundle("Config HW"=w5, "Config Test"=w6, "Config VGA"=w7, "CONFIG GEN"=w1) -> (w3:T18)  [unwired: 1 in]
  n5 = while {
    shift-right: [w14] -> w8
    shift-left: machine_estate_configs."Init" ("MACHINE") -> [w15]
    shift-right: [w12] -> _
    shift-left: w3 -> [w13]
    tunnel: "Path Config file" -> [w11]
    stop <- w16 stop-if-true
    n6 = case shown="\"wait\"" w15 {
      selector: w15 -> [_ _ _ _ _ _ _ _ w274 _ _ _]
      tunnel: [FALSE FALSE FALSE FALSE FALSE TRUE FALSE TRUE w275 FALSE FALSE FALSE] -> w16
      tunnel: [machine_estate_configs."load init file" ("MACHINE") machine_estate_configs."Test>View" ("MACHINE") machine_estate_configs."Test>View" ("MACHINE") machine_estate_configs."wait" ("MACHINE") machine_estate_configs."wait" ("MACHINE") machine_estate_configs."quit" ("MACHINE") machine_estate_configs."wait" ("MACHINE") machine_estate_configs."Init" ("MACHINE") w273 machine_estate_configs."wait" ("MACHINE") machine_estate_configs."Save File" ("MACHINE") machine_estate_configs."Valores>Test" ("MACHINE")] -> w14
      tunnel: [w43 w84 w96 w128 w236 w240 w244 w267 w271 w798 w879 w957] -> w12
      tunnel: w13 -> [w43 w87 w97 w128 w236 w240 w244 w267 w272 w799 w877 w957]
      tunnel: w11 -> [_ _ _ _ _ _ _ _ _ _ _ _]
      frame "Init", Default {
        w17 = FALSE  # algun cambio
        w20 = FALSE  # algun cambio
        w35 = "" ("CTA Test#")
        w54 = TRUE ("Front Panel Window:Show Menu Bar")
        n7 = control-ref of="visualize"() -> (w65:refnum<vi>)
        n8 = control-ref of="This VI"() -> (w51:refnum<vi>)
        n9 = control-ref of="Values Gen"() -> (w18:refnum<vi>)
        n10 = control-ref of="VALUES VGA"() -> (w22:refnum<vi>)
        n11 = Bundle("Column Headers"=string[] ["50 mV", "100 mV", "200 mV", "300 mV", "400 mV", "500 mV", "600 mV", "700 mV", "800 mV", "900 mV", "1000 mV"]) -> (w46:cluster{"Column Headers":string[]})  [unwired: 1 in]
        n12 = Bundle("Column Headers"=string[] ["REFP_0 (CH 00)", "REFC_0 (CH 01)", "REFN_0 (CH 02)", "IBIAST (CH 03)", "PTHT (CH 04)", "ADDOUT N (CH 05)", "ADDOUT P (CH 06)", "NTHT (CH 07)", "REFN_1 (CH 08)", "REFP_1 (CH 09)", "VCOM (CH 10)"]) -> (w55:cluster{"Column Headers":string[]})  [unwired: 1 in]
        n13 = Bundle("Column Headers"=string[] ["MAXIMUM P", "MINIMUM P", "MAXIMUM N", "MINIMUM N"]) -> (w56:cluster{"Column Headers":string[]})  [unwired: 1 in]
        n14 = Bundle("Column Headers"=string[] ["50 mV", "100 mV", "200 mV", "300 mV", "400 mV", "500 mV", "600 mV", "700 mV", "800 mV", "900 mV", "1000 mV"]) -> (w57:cluster{"Column Headers":string[]})  [unwired: 1 in]
        n15 = Bundle("Column Headers"=string[] ["50 mV (MODE 2)", "50 mV (MODE 3)", "50 mV (MODE 4)", "100 mV (MODE 2)", "100 mV (MODE 3)", "100 mV (MODE 4)", "200 mV (MODE 2)", "200 mV (MODE 3)", "200 mV (MODE 4)"]) -> (w58:cluster{"Column Headers":string[]})  [unwired: 1 in]
        n16 = control-ref of="LIMITS RATE SCAN ADDERS"() -> (w23:refnum<vi>)
        n17 = call "WINDOWS.AUTO SIZE.vi"("TAB.AutoAjuste"=w65, "This VI"=w51) -> ()  [unwired: 5 in, 1 out]
        n18 = control-ref of="LIMITS RATE SCAN"() -> (w24:refnum<vi>)
        n19 = control-ref of="LIMITS MAX PN MIN NP"() -> (w21:refnum<vi>)
        n20 = Bundle("Column Headers"=string[] ["CODE GAIN", "V REAL"]) -> (w44:cluster{"Column Headers":string[]})  [unwired: 1 in]
        n21 = control-ref of="LIMITS MEASUREMENT ADC"() -> (w25:refnum<vi>)
        n22 = Bundle("Column Headers"=string[] ["LOWER", "UPPER"]) -> (w49:cluster{"Column Headers":string[]})  [unwired: 1 in]
        n23 = property class="VI"(reference=w51, "Front Panel.ShowMenuBar"=w54, "TB.Visible"=w54, "Front Panel.TitleBarVis"=TRUE ("Front Panel Window:Title Bar Visible"), "Front Panel.Title"="CONFIG VALUES TEST" ("Front Panel Window:Title")) -> ()  [unwired: 1 in, 2 out]
        n24 = Build Array(w49, w49, w49, w49, w44) -> (w48:cluster{"Column Headers":string[]}[])
        n25 = Build Array(w55, w56, w57, w58, w46) -> (w63:cluster{"Column Headers":string[]}[])
        n26 = Build Array(w25, w21, w24, w23, w22, w18) -> (w64:refnum<vi>[])
        n27 = for {
          tunnel: w48 -> [w70] mode=indexing
          tunnel: w63 -> [w71] mode=indexing
          tunnel: w64 -> [w77] mode=indexing
          tunnel: [w68] -> w38
          w78 = FALSE ("Autosizing Row Height")
          w79 = TRUE ("Autosizing Row Height")
          n28 = Unbundle(w71) -> ("Column Headers"=w76:string[])
          n29 = Unbundle(w70) -> ("Column Headers"=w69:string[])
          n30 = Array Size(array=w69) -> (size(s)=w72:i32)
          n31 = Array Size(array=w76) -> (size(s)=w74:i32)
          n32 = Initialize Array("0", w74, w72) -> (w73:string[][])
          n33 = Increment(x=w74) -> (x+1=w80:i32)
          n34 = Increment(x=w72) -> (x+1=w81:i32)
          n35 = property on="Property Node" class="Tbl (strict)"(reference=w77, "Column Headers[]"=w69, "Number of Columns"=w81, "Row Headers[]"=w76, "Number of Rows"=w80, "Col Headers Vis"=w79, "Horizontal Lines Visible"=w79, "Horiz Scrollbar"=w78, "Index Visible"=w78, "Row Headers Vis"=w79, "Vertical Lines Visible"=w79, "Vert Scrollbar"=w78, "Val(Sgnl)"=w73) -> (error out=w68:errorcluster)  [unwired: 1 in, 1 out]
        }
        n36 = property on="Valores" class="Arr (strict)"("Index Values"=u32[] [0]) -> ()  [unwired: 2 in, 2 out]
        n37 = property on="vga test" class="Clust (strict)"("Visible"=FALSE) -> ()  [unwired: 2 in, 2 out]
        n38 = property on="VGA" class="Clust (strict)"("Visible"=TRUE) -> ()  [unwired: 2 in, 2 out]
        n39 = property on="QUIT" class="Bool"("DisabledEnum"=T19."Enabled" ("Disabled")) -> ()  [unwired: 2 in, 2 out]
        n40 = property on="Elemensts" class="LstBox (strict)"("EditRow"=0 ("Value (Signaling)"), "Item Names"=string[] []) -> ()  [unwired: 2 in, 2 out]
        n41 = local write "CHECK POWER"(FALSE ("CHECK POWER")) -> ()
        n42 = Bundle("CTA Test#"=w35, "CTA Test#"=w35) -> (w34:cluster{"CTA Test#":string, "CTA Test#":string})  [unwired: 1 in]
        n43 = local write "CHECK cta"(FALSE ("CHECK cta")) -> ()
        n44 = local write "CHECK vga"(FALSE ("CHECK vga")) -> ()
        n45 = property on="Valores" class="Arr (strict)"(error in=w38, "Value"=T16[] [] ("Valores")) -> ()  [unwired: 1 in, 2 out]
        n46 = Build Array(w34) -> (w33:T21)
        n47 = property on="Values Gen" class="Tbl (strict)"("Value"=string[][] [] ("VALUES VGA")) -> ()  [unwired: 2 in, 2 out]
        n48 = property on="VGA" class="Clust (strict)"("Value"=T2 {"VALUES VGA"=[], "TIME VGA"={"PULSE WIDTH"=0, "FRECUENCY PULSE"=0.0}} ("VGA")) -> ()  [unwired: 2 in, 2 out]
        n49 = property on="VISA Rigol DP832" class="VISAName"("Value"=refnum<visa-resource-name> refnum ("VISA Rigol DP832")) -> ()  [unwired: 2 in, 2 out]
        n50 = property on="Config Rigol DP832" class="Arr (strict)"("Value"=T15 [] ("Config Rigol DP832")) -> ()  [unwired: 2 in, 2 out]
        n51 = property on="CTA Board" class="CmbBox"("Strings And Values[]"=w33) -> ()  [unwired: 2 in, 2 out]
        "Cambios" <- w20
        "Primera llamada" <- w17
      }
      frame "load init file" {
        w83 = FALSE ("Cambios")
        n52 = local read "Path Config file"() -> (w82:path)
        n53 = Read from Text File(file (use dialog)=w82) -> (text=w89:string, error out=w88:errorcluster)  [unwired: 3 in, 2 out]
        n54 = Unflatten From XML(xml string=w89, type=w87, error in (no error)=w88) -> (value=w85:T18, error out=w86:errorcluster)
        n55 = case shown="Error" w86 {
          selector: w86 -> [_ w93]
          tunnel: w85 -> [w92 w94]
          tunnel: [w92 w94] -> w84
          frame No Error {
          }
          frame Error {
            n56 = call <vilib>:"Simple Error Handler.vi"("error in (no error)"=w93) -> ()  [unwired: 4 in, 5 out]
          }
        }
        n57 = local write "Primera llamada"(w83) -> ()
        n58 = local write "Cambios"(w83) -> ()
      }
      frame "Load File" {
        n59 = call <vilib>:"Application Directory.vi"() -> ("Application Directory"=w100:path)
        n60 = Build Path(base path=w100, name or relative path="Config") -> (appended path=w107:path)
        n61 = call <vilib>:"Check if File or Folder Exists.vi"("path"=w107) -> ("file or folder exists?"=w99:bool, "dup path"=w106:path)  [unwired: 8 in, 1 out]
        n62 = case shown="False" w99 {
          tunnel: w106 -> [w124 w125]
          tunnel: [w123 w125] -> w95
          frame False {
            n63 = Create Folder(path (use dialog)=w124) -> (created path=w123:path)  [unwired: 2 in, 2 out]
          }
          frame True {
          }
        }
        n64 = call "File Dialog2"("start path"=w95, "prompt"="Load Config TEST File", "button label"="Load", "pattern (all files)"="*.test", "pattern label"="Config files Test") -> ("selected path"=w102:path, "cancelled"=w101:bool, "error out"=w98:errorcluster)  [unwired: 7 in, 1 out]
        n65 = case shown="False" w101 {
          tunnel: w102 -> [w116 _]
          tunnel: w98 -> [_ _]
          tunnel: [w114 w122] -> w96
          tunnel: w97 -> [w117 w122]
          frame False {
            w112 = FALSE ("Cambios")
            n66 = local write "Path Config file"(w116) -> ()
            n67 = Read from Text File(file (use dialog)=w116) -> (text=w118:string)  [unwired: 3 in, 3 out]
            n68 = Unflatten From XML(xml string=w118, type=w117) -> (value=w113:T18, error out=w115:errorcluster)  [unwired: 1 in]
            n69 = local write "Cambios"(w112) -> ()
            n70 = local write "Primera llamada"(w112) -> ()
            n71 = case shown="Error" w115 {
              selector: w115 -> [_ w120]
              tunnel: [w119 w121] -> w114
              tunnel: w113 -> [w119 w121]
              frame No Error {
              }
              frame Error {
                n72 = call <vilib>:"Simple Error Handler.vi"("error in (no error)"=w120) -> ()  [unwired: 4 in, 5 out]
              }
            }
          }
          frame True {
          }
        }
      }
      frame "Test>View" {
        n73 = local read "Valores"() -> (w158:T16[])
        n74 = Unbundle By Name(w128) -> ("Config HW.VISA Key 81160A"=w129:refnum<visa-resource-name>, "Config HW.VISA Tek MDO3104"=w130:refnum<visa-resource-name>, "Config HW.VISA Rigol DP832"=w152:refnum<visa-resource-name>, "Config HW.CTA Test#"=w131:string)
        n75 = Unbundle By Name(w128) -> ("Config Test"=w155:T6)
        n76 = Unbundle By Name(w128) -> ("Config HW.Config Rigol DP832"=w139:T15)
        n77 = Unbundle By Name(w128) -> ("Config VGA.Real Voltage"=w143:dbl[], "Config VGA.VGA Gain"=w142:u8[], "Config VGA.Pulse Width"=w149:u16, "Config VGA.Frecuency Pulse"=w150:dbl)
        n78 = Unbundle By Name(w128) -> ("CONFIG GEN"=w126:T1[])
        "CONFIG GEN temp" <- w126
        n79 = Index Array(array=w158, index=0) -> (element=w157:T16)
        n80 = for {
          tunnel: w157 -> [w235]
          tunnel: w155 -> [w234] mode=indexing
          tunnel: [w194] -> w153 mode=indexing
          tunnel: [w179] -> w136 mode=indexing
          n81 = Unbundle By Name(w234) -> ("Vasic"=w182:dbl, "Vasic real f.a."=w177:dbl, "Global Reset"=w178:bool, "IBIAS"=w176:bool, "VALUE IBIAS"=w175:u8, "Test Register?"=w193:bool, "Test ADC?"=w233:bool, "Test ADC.Repeats ADC"=w232:i32, "Test ADC.Max Desviation"=w231:dbl, "Limits ADC.Low"=w220:dbl[], "Limits ADC.High"=w219:dbl[], "Test Max PN Min NP?"=w230:bool, "Limits Max PN Min NP.Max P Upper"=w192:dbl, "Limits Max PN Min NP.Min P Upper"=w191:dbl, "Limits Max PN Min NP.Max N Upper"=w190:dbl, "Limits Max PN Min NP.Min N Upper"=w189:dbl, "Limits Max PN Min NP.Max P Lower"=w186:dbl, "Limits Max PN Min NP.Min P Lower"=w185:dbl, "Limits Max PN Min NP.Max N Lower"=w184:dbl, "Limits Max PN Min NP.Min N Lower"=w183:dbl, "Test Rate Scan?"=w212:bool, "Vin Rate Scan"=w211:i32[], "Limits Rate Scan.High"=w202:dbl[], "Limits Rate Scan.Low"=w201:dbl[], "Test Rate Scan Adders?"=w195:bool, "Vin Rate Adders"=w198:i32[], "Limits Rate Scan adders.High"=w200:dbl[], "Limits Rate Scan adders.Low"=w199:dbl[], "Test offset analog?"=w225:bool, "Lim Offset Analog.Max Analog"=w226:dbl, "Lim Offset Analog.Min Analog"=w227:dbl, "Test offset digital?"=w228:bool, "Lim offset Dig.Max Dig"=w229:dbl)
          n82 = Build Array(w220, w219) -> (w222:dbl[][])
          n83 = Build Array(w199, w200) -> (w205:dbl[][])
          n84 = Build Array(w201, w202) -> (w208:dbl[][])
          n85 = Build Array(w192, w191, w190, w189) -> (w188:dbl[])
          n86 = Build Array(w186, w185, w184, w183) -> (w187:dbl[])
          n87 = Transpose 2D Array(2D array=w222) -> (transposed array=w221:dbl[][])
          n88 = Transpose 2D Array(2D array=w208) -> (transposed array=w207:dbl[][])
          n89 = Transpose 2D Array(2D array=w205) -> (transposed array=w206:dbl[][])
          n90 = Build Array(w187, w188) -> (w216:dbl[][])
          n91 = Transpose 2D Array(2D array=w216) -> (transposed array=w217:dbl[][])
          n92 = Number To Fractional String(number=w221, width (-)=i16 1, precision (6)=i16 4) -> (F-format string=w218:string[][])  [unwired: 1 in]
          n93 = Number To Fractional String(number=w207, width (-)=i16 1, precision (6)=i16 4) -> (F-format string=w196:string[][])  [unwired: 1 in]
          n94 = Number To Fractional String(number=w206, width (-)=i16 1, precision (6)=i16 4) -> (F-format string=w197:string[][])  [unwired: 1 in]
          n95 = Number To Fractional String(number=w217, width (-)=i16 1, precision (6)=i16 4) -> (F-format string=w213:string[][])  [unwired: 1 in]
          n96 = Bundle By Name(cluster=w235, "VOLTAGE SUPPLY ASIC"=w182, "V SUPPLY ASIC REAL"=w177, "GLOBAL RESET"=w178, "IBIAS"=w176, "VALUE IBIAS"=w175, "TEST REGISTER"=w193, "TEST ADC"=w233, "SETUP ADC.NUMBER OF REPETITIONS"=w232, "SETUP ADC.MAX DESVIATION ADC"=w231, "LIMITS MEASUREMENT ADC"=w218, "TEST MAX MIN P/N"=w230, "LIMITS MAX PN MIN NP"=w213, "TEST RATE SCAN"=w212, "VIN ASIC"=w211, "LIMITS RATE SCAN"=w196, "TEST RATE SCAN ADDERS"=w195, "VIN ASIC ADD"=w198, "LIMITS RATE SCAN ADDERS"=w197, "TEST OFFSET ANALOG"=w225, "LIMITS OFFSET ANALOG.MAXIMUM"=w226, "LIMITS OFFSET ANALOG.MINIMUM"=w227, "TEST OFFSET DIGITAL"=w228, "LIMITS OFFSET DIGITAL.MAXIMUM"=w229) -> (w194:T16)
          n97 = Number To Fractional String(number=w182, width (-)=i16 1, precision (6)=i16 2) -> (F-format string=w179:string)  [unwired: 1 in]
        }
        n98 = for {
          tunnel: w126 -> [w174] mode=indexing
          tunnel: [w161] -> w127 mode=indexing
          n99 = Unbundle By Name(w174) -> ("Amplitude"=w172:dbl, "Frequency"=w166:dbl, "Width Time"=w167:dbl, "Load"=w168:dbl)
          n100 = Format Value(format string="%#_6pHz", value (0)=w166) -> (output string=w164:string)  [unwired: 1 in]
          n101 = Format Value(format string="%#_6pV", value (0)=w172) -> (output string=w165:string)  [unwired: 1 in]
          n102 = Format Value(format string="%#_6ps", value (0)=w167) -> (output string=w163:string)  [unwired: 1 in]
          n103 = Format Value(format string="%#_6pOhm", value (0)=w168) -> (output string=w162:string)  [unwired: 1 in]
          n104 = Build Array(w165, w164, w163, w162) -> (w161:string[])
        }
        n105 = Number To Fractional String(number=w143, width (-)=i16 1, precision (6)=i16 4) -> (F-format string=w144:string[])  [unwired: 1 in]
        n106 = Bundle("CTA Test#"=w131, "CTA Test#"=w131) -> (w138:cluster{"CTA Test#":string, "CTA Test#":string})  [unwired: 1 in]
        n107 = property on="Config Rigol DP832" class="Arr (strict)"("Value"=w139) -> ()  [unwired: 2 in, 2 out]
        n108 = property on="VISA Generator Key 81160A" class="VISAName"("Value"=w129) -> ()  [unwired: 2 in, 2 out]
        n109 = property on="VISA Oscilloscope Tek MDO3104" class="VISAName"("Value"=w130) -> ()  [unwired: 2 in, 2 out]
        n110 = property on="VISA Rigol DP832" class="VISAName"("Value"=w152) -> ()  [unwired: 2 in, 2 out]
        n111 = Build Array(w138) -> (w137:T21)
        n112 = Number To Decimal String(number=w142) -> (decimal integer string=w145:string[])  [unwired: 1 in]
        n113 = Build Array(w145, w144) -> (w146:string[][])
        n114 = property on="CTA Board" class="CmbBox"("Strings And Values[]"=w137) -> (error out=w132:errorcluster)  [unwired: 2 in, 1 out]
        n115 = Transpose 2D Array(2D array=w146) -> (transposed array=w141:string[][])
        n116 = property on="Values Gen" class="Tbl (strict)"("Value"=w127) -> ()  [unwired: 2 in, 2 out]
        n117 = property on="CTA Board" class="CmbBox"(error in=w132, "Value"=w131) -> ()  [unwired: 1 in, 2 out]
        n118 = local read "VGA"() -> (w151:T2)
        n119 = Bundle By Name(cluster=w151, "VALUES VGA"=w141, "TIME VGA.PULSE WIDTH"=w149, "TIME VGA.FRECUENCY PULSE"=w150) -> (w140:T2)
        n120 = property on="Valores" class="Arr (strict)"() -> ("Index Values"=w135:u32[])  [unwired: 2 in, 2 out]
        n121 = property on="VGA" class="Clust (strict)"("Value"=w140) -> ()  [unwired: 2 in, 2 out]
        n122 = Index Array(array=w135, index=0) -> (element=w134:u32)
        n123 = property on="Elemensts" class="LstBox (strict)"("EditRow"=w134, "Item Names"=w136) -> ()  [unwired: 2 in, 2 out]
        n124 = property on="Valores" class="Arr (strict)"("Value"=w153) -> (error out=w154:errorcluster)  [unwired: 2 in, 1 out]
        n125 = property on="Valores" class="Arr (strict)"(error in=w154, "Val(Sgnl)"=w153) -> ()  [unwired: 1 in, 2 out]
      }
      frame "Refresh" {
      }
      frame "quit" {
        n126 = local write "Cambios"(FALSE ("Cambios")) -> ()
      }
      frame "Save File" {
        n127 = call <vilib>:"Application Directory.vi"() -> ("Application Directory"=w247:path)
        n128 = Build Path(base path=w247, name or relative path="Config") -> (appended path=w255:path)
        n129 = call <vilib>:"Check if File or Folder Exists.vi"("path"=w255) -> ("file or folder exists?"=w246:bool, "dup path"=w254:path)  [unwired: 8 in, 1 out]
        n130 = case shown="True" w246 {
          tunnel: w254 -> [w264 w265]
          tunnel: [w263 w265] -> w253
          frame False {
            n131 = Create Folder(path (use dialog)=w264) -> (created path=w263:path)  [unwired: 2 in, 2 out]
          }
          frame True {
          }
        }
        n132 = call "File Dialog"("start path"=w253, "prompt"="Save Config TEST File", "button label"="Save", "pattern (all files)"="*.test", "pattern label"="Config files Test") -> ("selected path"=w249:path, "cancelled"=w248:bool, "error out"=w245:errorcluster)  [unwired: 7 in, 1 out]
        n133 = case shown="False" w248 {
          tunnel: w249 -> [w262 _]
          tunnel: w245 -> [_ _]
          tunnel: w244 -> [w261 _]
          frame False {
            n134 = Flatten To XML(anything=w261) -> (xml string=w260:string)
            n135 = local write "Path Config file"(w262) -> ()
            n136 = local write "Cambios"(FALSE ("Cambios")) -> ()
            n137 = Write to Text File(file (use dialog)=w262, text=w260) -> ()  [unwired: 2 in, 3 out]
          }
          frame True {
          }
        }
      }
      frame "quit save" {
        n138 = local write "Cambios"(FALSE ("Cambios")) -> ()
      }
      frame "wait" {
        n139 = event shown="[16] \"Change value Gen\": Value Change" {
          selector: _ -> [_ _ _ _ _ _ _ _ _ _ _ _ _ _ _ _ _ _ _]
          dyn-events: _ -> [_ _ _ _ _ _ _ _ _ _ _ _ _ _ _ _ _ _ _]
          timeout: 1000 -> [_ _ _ _ _ _ _ _ _ _ _ _ _ _ _ _ _ _ _]
          tunnel: [FALSE FALSE FALSE FALSE FALSE FALSE FALSE FALSE FALSE FALSE FALSE FALSE FALSE FALSE FALSE FALSE FALSE w762 FALSE] -> w275
          tunnel: w274 -> [_ _ _ _ _ _ _ _ _ _ _ _ _ _ _ _ _ _ _]
          tunnel: [machine_estate_configs."wait" ("MACHINE") machine_estate_configs."Valores>Test" ("MACHINE") w317 machine_estate_configs."wait" ("MACHINE") machine_estate_configs."Valores>Test" ("MACHINE") machine_estate_configs."wait" ("MACHINE") machine_estate_configs."wait" ("MACHINE") machine_estate_configs."Valores>Test" ("MACHINE") machine_estate_configs."Valores>Test" ("MACHINE") w653 machine_estate_configs."wait" ("MACHINE") machine_estate_configs."wait" ("MACHINE") machine_estate_configs."wait" ("MACHINE") machine_estate_configs."wait" ("MACHINE") machine_estate_configs."wait" ("MACHINE") machine_estate_configs."wait" ("MACHINE") machine_estate_configs."wait" ("MACHINE") w761 machine_estate_configs."Save In Config" ("MACHINE")] -> w273
          tunnel: w272 -> [w277 w293 w318 w328 w393 w471 w552 w563 w586 w655 w684 w698 _ _ _ _ w735 w763 w784]
          tunnel: [w277 w293 w318 w328 w393 w471 w552 w563 w586 w655 w684 w698 _ _ _ _ w735 w763 w784] -> w271
          event Timeout {
            # "Chapuza para evitar la pregunta en quit"
            n140 = event-data() -> ()  [unwired: 1 in, 2 out]
            n141 = local read "Primera llamada"() -> (w276:bool)
            n142 = case shown="True" w276 {
              frame False {
                n143 = local write "Cambios"(FALSE ("Cambios")) -> ()
                n144 = local write "Primera llamada"(TRUE ("Primera llamada")) -> ()
              }
              frame True {
              }
            }
          }
          event "Valores": Value Change {
            n145 = event-data() -> ("OldVal"=w294:T16[], "NewVal"=w283:T16[])  [unwired: 1 in, 3 out]
            n146 = Array Size(array=w283) -> (size(s)=w284:i32)
            n147 = for {
              N: w284 -> [_]
              tunnel: w283 -> [w303] mode=indexing
              tunnel: w294 -> [w314] mode=indexing
              tunnel: [w311] -> w288 mode=indexing
              n148 = Unbundle By Name(w303) -> ("LIMITS MEASUREMENT ADC"=w310:string[][], "LIMITS MAX PN MIN NP"=w308:string[][], "LIMITS RATE SCAN"=w304:string[][], "LIMITS RATE SCAN ADDERS"=w305:string[][])
              n149 = Unbundle By Name(w314) -> ("LIMITS MEASUREMENT ADC"=w313:string[][], "LIMITS MAX PN MIN NP"=w309:string[][], "LIMITS RATE SCAN"=w307:string[][], "LIMITS RATE SCAN ADDERS"=w306:string[][])
              n150 = call "GUI.Comprueba limites.vi"("LIMITS MEASUREMENT ADC"=w310, "LIMITS MEASUREMENT ADC 2"=w313) -> ("Array"=w312:string[][])
              n151 = call "GUI.Comprueba limites.vi"("LIMITS MEASUREMENT ADC"=w308, "LIMITS MEASUREMENT ADC 2"=w309) -> ("Array"=w302:string[][])
              n152 = call "GUI.Comprueba limites.vi"("LIMITS MEASUREMENT ADC"=w304, "LIMITS MEASUREMENT ADC 2"=w307) -> ("Array"=w301:string[][])
              n153 = call "GUI.Comprueba limites.vi"("LIMITS MEASUREMENT ADC"=w305, "LIMITS MEASUREMENT ADC 2"=w306) -> ("Array"=w300:string[][])
              n154 = Bundle By Name(cluster=w303, "LIMITS MEASUREMENT ADC"=w312, "LIMITS MAX PN MIN NP"=w302, "LIMITS RATE SCAN"=w301, "LIMITS RATE SCAN ADDERS"=w300) -> (w311:T16)
            }
            n155 = First Call?() -> (First Call?: T/F=w282:bool)
            n156 = for {
              tunnel: [w299] -> w289 mode=indexing
              tunnel: w288 -> [w298] mode=indexing
              n157 = Unbundle By Name(w298) -> ("VOLTAGE SUPPLY ASIC"=w299:dbl)
            }
            n158 = property on="Valores" class="Arr (strict)"() -> ("Index Values"=w287:u32[])  [unwired: 2 in, 2 out]
            n159 = case shown="False" w282 {
              frame False {
                n160 = local write "Cambios"(TRUE ("Cambios")) -> ()
              }
              frame True {
              }
            }
            n161 = Index Array(array=w287, index=0) -> (element=w285:u32)
            n162 = Number To Fractional String(number=w289, width (-)=i16 1, precision (6)=i16 2) -> (F-format string=w290:string[])  [unwired: 1 in]
            n163 = property on="Elemensts" class="LstBox (strict)"("Value"=w285, "EditRow"=w285, "Item Names"=w290) -> ()  [unwired: 2 in, 2 out]
            n164 = local write "Valores"(w288) -> ()
          }
          event "default": Value Change {
            n165 = event-data() -> ()  [unwired: 1 in, 5 out]
            n166 = local read "Cambios"() -> (w316:bool)
            n167 = case shown="False" w316 {
              tunnel: [machine_estate_configs."Default values" ("MACHINE") w320] -> w317
              frame False {
              }
              frame True {
                n168 = call "Display Message to User2"() -> ("Don't Save & Load Default"=w323:bool)  [unwired: 10 in, 1 out]
                n169 = Select(t=machine_estate_configs."Default values" ("MACHINE"), s=w323, f=machine_estate_configs."wait" ("MACHINE")) -> (s? t:f=w320:T17)
              }
            }
          }
          event "CHECK POWER": Value Change {
            n170 = local read "Config Rigol DP832"() -> (w325:T15)
            n171 = event-data() -> ()  [unwired: 1 in, 5 out]
            n172 = local read "VISA Rigol DP832"() -> (w326:refnum<visa-resource-name>)
            n173 = case shown="True" "CHECK POWER" {
              tunnel: w326 -> [w335 w359]
              tunnel: w325 -> [w334 w358]
              frame False {
                n174 = call "DP832_Enable ALL Output.vi"("Enable Output (T: Enable)"=FALSE, "error in (no error)"=errorcluster {"status"=FALSE, "code"=0, "source"=""}, "VISA resource name"=w335) -> ("error out"=w340:errorcluster, "VISA resource name out"=w341:refnum<visa-resource-name>)  [unwired: 7 in]
                n175 = for {
                  shift-right: [w349] -> w336
                  shift-left: w340 -> [w345]
                  shift-right: [w350] -> w337
                  shift-left: w341 -> [w346]
                  tunnel: w334 -> [w344] mode=indexing
                  w343 = 0.0  # Voltage Level
                  w347 = 0.0  # Current Limit
                  w351 = T22 0 items=["Regulate", "Trip"] ("Behavior (0: Regulate)")
                  n176 = Unbundle By Name(w344) -> ("Channel"=w348:T5)
                  n177 = call "DP832_Configure Current Limit.vi"("Behavior"=w351, "error in (no error)"=w345, "Current Limit"=w347, "Channel"=w348, "VISA resource name"=w346) -> ("error out"=w353:errorcluster, "VISA resource name out"=w354:refnum<visa-resource-name>)  [unwired: 5 in]
                  n178 = call "DP832_Configure Output.vi"("Enable Output (T: Enable)"=FALSE, "error in (no error)"=w353, "Voltage Level"=w343, "Channel"=w348, "VISA resource name"=w354) -> ("error out"=w349:errorcluster, "VISA resource name out"=w350:refnum<visa-resource-name>)  [unwired: 5 in]
                }
                n179 = call "DP832_Local Mode.vi"("error in (no error)"=w336, "VISA resource name"=w337) -> ("error out"=w339:errorcluster, "VISA resource name out"=w338:refnum<visa-resource-name>)  [unwired: 8 in]
                n180 = call "DP832_Close.vi"("error in (no error)"=w339, "VISA resource name"=w338) -> ("error out"=w332:errorcluster)  [unwired: 8 in, 1 out]
                n181 = call <vilib>:"Clear Errors.vi"("error in (no error)"=w332) -> ("error out"=w330:errorcluster)  [unwired: 5 in, 1 out]
                n182 = property on="QUIT" class="Bool"(error in=w330, "DisabledEnum"=T19."Enabled" ("Disabled")) -> ()  [unwired: 1 in, 2 out]
              }
              frame True {
                w355 = errorcluster {"status"=FALSE, "code"=0, "source"=""} ("error in")
                n183 = for {
                  N: 3 -> [_]
                  tunnel: [w364] -> w357
                  tunnel: w358 -> [w370]
                  tunnel: w359 -> [w367]
                  tunnel: w355 -> [w366]
                  stop <- w362 continue-if-true
                  n184 = call "Prueba_rigol.vi"("error in (no error)"=w366, "VISA IN"=w367) -> ("error out 2"=w365:errorcluster)  [unwired: 8 in, 1 out]
                  n185 = call "DP832_Init gustavo.vi"("error in (no error)"=w365, "VISA resource name 2"=w367) -> ("error out"=w368:errorcluster, "VISA resource name"=w369:refnum<visa-resource-name>)
                  n186 = call "DP832_Beep.vi"("error in (no error)"=w368, "VISA resource name"=w369) -> ("error out"=w374:errorcluster, "VISA resource name out"=w375:refnum<visa-resource-name>)  [unwired: 8 in]
                  n187 = for {
                    shift-right: [w381] -> w372
                    shift-left: w374 -> [w383]
                    shift-right: [w382] -> w373
                    shift-left: w375 -> [w384]
                    tunnel: w370 -> [w380] mode=indexing
                    w385 = T22 0 items=["Regulate", "Trip"] ("Behavior (0: Regulate)")
                    n188 = Unbundle By Name(w380) -> ("Channel"=w378:T5, "V Limit"=w379:dbl, "I Limit"=w377:dbl, "V Out"=w376:dbl)
                    n189 = call "DP832_Configure OVP.vi"("Enable OVP (T: Enable)"=FALSE, "error in (no error)"=w383, "Voltage Limit"=w379, "Channel"=w378, "VISA resource name"=w384) -> ("error out"=w388:errorcluster, "VISA resource name out"=w387:refnum<visa-resource-name>)  [unwired: 5 in]
                    n190 = call "DP832_Configure Current Limit.vi"("Behavior"=w385, "error in (no error)"=w388, "Current Limit"=w377, "Channel"=w378, "VISA resource name"=w387) -> ("error out"=w390:errorcluster, "VISA resource name out"=w391:refnum<visa-resource-name>)  [unwired: 5 in]
                    n191 = call "DP832_Configure Output.vi"("Enable Output (T: Enable)"=FALSE, "error in (no error)"=w390, "Voltage Level"=w376, "Channel"=w378, "VISA resource name"=w391) -> ("error out"=w381:errorcluster, "VISA resource name out"=w382:refnum<visa-resource-name>)  [unwired: 5 in]
                  }
                  n192 = call "DP832_Enable ALL Output.vi"("Enable Output (T: Enable)"=TRUE, "error in (no error)"=w372, "VISA resource name"=w373) -> ("error out"=w364:errorcluster)  [unwired: 7 in, 1 out]
                  n193 = Select(t=TRUE, s=w364, f=FALSE) -> (s? t:f=w362:bool)
                }
                n194 = property on="QUIT" class="Bool"(error in=w355, "DisabledEnum"=T19."Disabled and Grayed Out" ("Disabled")) -> ()  [unwired: 1 in, 2 out]
                n195 = call <vilib>:"Clear Errors.vi"("error in (no error)"=w357) -> ()  [unwired: 5 in, 2 out]
              }
            }
          }
          event "CHECK cta": Value Change {
            n196 = event-data() -> ()  [unwired: 1 in, 5 out]
            n197 = local read "Config Rigol DP832"() -> (w397:T15)
            n198 = local read "VISA Rigol DP832"() -> (w396:refnum<visa-resource-name>)
            n199 = case shown="True" "CHECK cta" {
              tunnel: w396 -> [w401 w433]
              tunnel: w397 -> [w400 w432]
              frame False {
                w399 = errorcluster {"status"=FALSE, "code"=0, "source"=""} ("error in")
                n200 = call "DP832_Enable ALL Output.vi"("Enable Output (T: Enable)"=FALSE, "error in (no error)"=w399, "VISA resource name"=w401) -> ("error out"=w406:errorcluster, "VISA resource name out"=w407:refnum<visa-resource-name>)  [unwired: 7 in]
                n201 = for {
                  shift-right: [w416] -> w402
                  shift-left: w406 -> [w412]
                  shift-right: [w417] -> w403
                  shift-left: w407 -> [w413]
                  tunnel: w400 -> [w411] mode=indexing
                  w410 = 0.0  # Voltage Level
                  w414 = 0.0  # Current Limit
                  w418 = T22 0 items=["Regulate", "Trip"] ("Behavior (0: Regulate)")
                  n202 = Unbundle By Name(w411) -> ("Channel"=w415:T5)
                  n203 = call "DP832_Configure Current Limit.vi"("Behavior"=w418, "error in (no error)"=w412, "Current Limit"=w414, "Channel"=w415, "VISA resource name"=w413) -> ("error out"=w420:errorcluster, "VISA resource name out"=w421:refnum<visa-resource-name>)  [unwired: 5 in]
                  n204 = call "DP832_Configure Output.vi"("Enable Output (T: Enable)"=FALSE, "error in (no error)"=w420, "Voltage Level"=w410, "Channel"=w415, "VISA resource name"=w421) -> ("error out"=w416:errorcluster, "VISA resource name out"=w417:refnum<visa-resource-name>)  [unwired: 5 in]
                }
                n205 = flat-sequence {
                  tunnel: w399 -> [_]
                  frame #0 {
                    n206 = local read "FT_Handle"() -> (w409:u32)
                    n207 = call "FT_Close_Device.vi"("Handle"=w409) -> ()  [unwired: 1 out]
                  }
                }
                n208 = call "DP832_Local Mode.vi"("error in (no error)"=w402, "VISA resource name"=w403) -> ("error out"=w405:errorcluster, "VISA resource name out"=w404:refnum<visa-resource-name>)  [unwired: 8 in]
                n209 = call "DP832_Close.vi"("error in (no error)"=w405, "VISA resource name"=w404) -> ("error out"=w398:errorcluster)  [unwired: 8 in, 1 out]
                n210 = call <vilib>:"Clear Errors.vi"("error in (no error)"=w398) -> ()  [unwired: 5 in, 2 out]
              }
              frame True {
                n211 = property on="CTA Board" class="CmbBox"() -> ("Value"=w427:string)  [unwired: 2 in, 2 out]
                n212 = for {
                  N: 3 -> [_]
                  tunnel: [w442] -> w431
                  tunnel: w432 -> [w448]
                  tunnel: w433 -> [w445]
                  tunnel: errorcluster {"status"=FALSE, "code"=0, "source"=""} ("error in") -> [w444]
                  stop <- w440 continue-if-true
                  n213 = call "Prueba_rigol.vi"("error in (no error)"=w444, "VISA IN"=w445) -> ("error out 2"=w443:errorcluster)  [unwired: 8 in, 1 out]
                  n214 = call "DP832_Init gustavo.vi"("error in (no error)"=w443, "VISA resource name 2"=w445) -> ("error out"=w446:errorcluster, "VISA resource name"=w447:refnum<visa-resource-name>)
                  n215 = call "DP832_Beep.vi"("error in (no error)"=w446, "VISA resource name"=w447) -> ("error out"=w452:errorcluster, "VISA resource name out"=w453:refnum<visa-resource-name>)  [unwired: 8 in]
                  n216 = for {
                    shift-right: [w459] -> w450
                    shift-left: w452 -> [w461]
                    shift-right: [w460] -> w451
                    shift-left: w453 -> [w462]
                    tunnel: w448 -> [w458] mode=indexing
                    w463 = T22 0 items=["Regulate", "Trip"] ("Behavior (0: Regulate)")
                    n217 = Unbundle By Name(w458) -> ("Channel"=w456:T5, "V Limit"=w457:dbl, "I Limit"=w455:dbl, "V Out"=w454:dbl)
                    n218 = call "DP832_Configure OVP.vi"("Enable OVP (T: Enable)"=FALSE, "error in (no error)"=w461, "Voltage Limit"=w457, "Channel"=w456, "VISA resource name"=w462) -> ("error out"=w466:errorcluster, "VISA resource name out"=w465:refnum<visa-resource-name>)  [unwired: 5 in]
                    n219 = call "DP832_Configure Current Limit.vi"("Behavior"=w463, "error in (no error)"=w466, "Current Limit"=w455, "Channel"=w456, "VISA resource name"=w465) -> ("error out"=w468:errorcluster, "VISA resource name out"=w469:refnum<visa-resource-name>)  [unwired: 5 in]
                    n220 = call "DP832_Configure Output.vi"("Enable Output (T: Enable)"=FALSE, "error in (no error)"=w468, "Voltage Level"=w454, "Channel"=w456, "VISA resource name"=w469) -> ("error out"=w459:errorcluster, "VISA resource name out"=w460:refnum<visa-resource-name>)  [unwired: 5 in]
                  }
                  n221 = call "DP832_Enable ALL Output.vi"("Enable Output (T: Enable)"=TRUE, "error in (no error)"=w450, "VISA resource name"=w451) -> ("error out"=w442:errorcluster)  [unwired: 7 in, 1 out]
                  n222 = Select(t=TRUE, s=w442, f=FALSE) -> (s? t:f=w440:bool)
                }
                n223 = call <vilib>:"Clear Errors.vi"("error in (no error)"=w431) -> ("error out"=w423:errorcluster)  [unwired: 5 in, 1 out]
                n224 = call "FT_Search All Select description.vi"("error in (no error)"=w423, "CTA Test#"=w427) -> ("error Out"=w422:errorcluster, "All FT"=w428:T23, "Select Ft"=w430:T24)  [unwired: 7 in]
                n225 = call <vilib>:"Clear Errors.vi"("error in (no error)"=w422) -> ()  [unwired: 5 in, 2 out]
                n226 = for {
                  tunnel: w428 -> [w438] mode=indexing
                  tunnel: [w436] -> w426 mode=indexing
                  n227 = Unbundle By Name(w438) -> ("Serial Number"=w437:string)
                  n228 = Bundle("Serial Number"=w437, "Serial Number"=w437) -> (w436:T25)  [unwired: 1 in]
                }
                n229 = Unbundle By Name(w430) -> ("FT_Handle"=→"FT_Handle":u32)
                n230 = property on="CTA Board" class="CmbBox"("Strings And Values[]"=w426) -> (error out=w424:errorcluster)  [unwired: 2 in, 1 out]
                n231 = property on="CHECK cta" class="Bool (strict)"(error in=w424, "Val(Sgnl)"=FALSE) -> ()  [unwired: 1 in, 2 out]
              }
            }
          }
          event "CHECK vga": Value Change {
            n232 = event-data() -> ()  [unwired: 1 in, 5 out]
            n233 = local read "Config Rigol DP832"() -> (w475:T15)
            n234 = local read "VISA Rigol DP832"() -> (w474:refnum<visa-resource-name>)
            n235 = case shown="True" "CHECK vga" {
              tunnel: w474 -> [w478 w510]
              tunnel: w475 -> [w477 w505]
              frame False {
                w476 = errorcluster {"status"=FALSE, "code"=0, "source"=""} ("error in")
                n236 = call "DP832_Enable ALL Output.vi"("Enable Output (T: Enable)"=FALSE, "error in (no error)"=w476, "VISA resource name"=w478) -> ("error out"=w483:errorcluster, "VISA resource name out"=w484:refnum<visa-resource-name>)  [unwired: 7 in]
                n237 = flat-sequence {
                  tunnel: w476 -> [_]
                  frame #0 {
                    n238 = property on="VGA" class="Clust (strict)"("Visible"=TRUE) -> ()  [unwired: 2 in, 2 out]
                    n239 = local read "FT_Handle"() -> (w489:u32)
                    n240 = property on="QUIT" class="Bool"("DisabledEnum"=T19."Enabled" ("Disabled")) -> ()  [unwired: 2 in, 2 out]
                    n241 = call "FT_Close_Device.vi"("Handle"=w489) -> ()  [unwired: 1 out]
                    n242 = property on="vga test" class="Clust (strict)"("Visible"=FALSE) -> ()  [unwired: 2 in, 2 out]
                  }
                }
                n243 = for {
                  shift-right: [w496] -> w479
                  shift-left: w483 -> [w492]
                  shift-right: [w497] -> w480
                  shift-left: w484 -> [w493]
                  tunnel: w477 -> [w491] mode=indexing
                  w490 = 0.0  # Voltage Level
                  w494 = 0.0  # Current Limit
                  w498 = T22 0 items=["Regulate", "Trip"] ("Behavior (0: Regulate)")
                  n244 = Unbundle By Name(w491) -> ("Channel"=w495:T5)
                  n245 = call "DP832_Configure Current Limit.vi"("Behavior"=w498, "error in (no error)"=w492, "Current Limit"=w494, "Channel"=w495, "VISA resource name"=w493) -> ("error out"=w500:errorcluster, "VISA resource name out"=w501:refnum<visa-resource-name>)  [unwired: 5 in]
                  n246 = call "DP832_Configure Output.vi"("Enable Output (T: Enable)"=FALSE, "error in (no error)"=w500, "Voltage Level"=w490, "Channel"=w495, "VISA resource name"=w501) -> ("error out"=w496:errorcluster, "VISA resource name out"=w497:refnum<visa-resource-name>)  [unwired: 5 in]
                }
                n247 = call "DP832_Local Mode.vi"("error in (no error)"=w479, "VISA resource name"=w480) -> ("error out"=w482:errorcluster, "VISA resource name out"=w481:refnum<visa-resource-name>)  [unwired: 8 in]
                n248 = call "DP832_Close.vi"("error in (no error)"=w482, "VISA resource name"=w481) -> ()  [unwired: 8 in, 2 out]
              }
              frame True {
                w502 = errorcluster {"status"=FALSE, "code"=0, "source"=""} ("error in")
                n249 = property on="CTA Board" class="CmbBox"() -> ("Value"=w507:string)  [unwired: 2 in, 2 out]
                n250 = for {
                  N: 3 -> [_]
                  tunnel: [w523] -> w509
                  tunnel: w505 -> [w529]
                  tunnel: w510 -> [w526]
                  tunnel: w502 -> [w525]
                  stop <- w521 continue-if-true
                  n251 = call "Prueba_rigol.vi"("error in (no error)"=w525, "VISA IN"=w526) -> ("error out 2"=w524:errorcluster)  [unwired: 8 in, 1 out]
                  n252 = call "DP832_Init gustavo.vi"("error in (no error)"=w524, "VISA resource name 2"=w526) -> ("error out"=w527:errorcluster, "VISA resource name"=w528:refnum<visa-resource-name>)
                  n253 = call "DP832_Beep.vi"("error in (no error)"=w527, "VISA resource name"=w528) -> ("error out"=w533:errorcluster, "VISA resource name out"=w534:refnum<visa-resource-name>)  [unwired: 8 in]
                  n254 = for {
                    shift-right: [w540] -> w531
                    shift-left: w533 -> [w542]
                    shift-right: [w541] -> w532
                    shift-left: w534 -> [w543]
                    tunnel: w529 -> [w539] mode=indexing
                    w544 = T22 0 items=["Regulate", "Trip"] ("Behavior (0: Regulate)")
                    n255 = Unbundle By Name(w539) -> ("Channel"=w537:T5, "V Limit"=w538:dbl, "I Limit"=w536:dbl, "V Out"=w535:dbl)
                    n256 = call "DP832_Configure OVP.vi"("Enable OVP (T: Enable)"=FALSE, "error in (no error)"=w542, "Voltage Limit"=w538, "Channel"=w537, "VISA resource name"=w543) -> ("error out"=w547:errorcluster, "VISA resource name out"=w546:refnum<visa-resource-name>)  [unwired: 5 in]
                    n257 = call "DP832_Configure Current Limit.vi"("Behavior"=w544, "error in (no error)"=w547, "Current Limit"=w536, "Channel"=w537, "VISA resource name"=w546) -> ("error out"=w549:errorcluster, "VISA resource name out"=w550:refnum<visa-resource-name>)  [unwired: 5 in]
                    n258 = call "DP832_Configure Output.vi"("Enable Output (T: Enable)"=FALSE, "error in (no error)"=w549, "Voltage Level"=w535, "Channel"=w537, "VISA resource name"=w550) -> ("error out"=w540:errorcluster, "VISA resource name out"=w541:refnum<visa-resource-name>)  [unwired: 5 in]
                  }
                  n259 = call "DP832_Enable ALL Output.vi"("Enable Output (T: Enable)"=TRUE, "error in (no error)"=w531, "VISA resource name"=w532) -> ("error out"=w523:errorcluster)  [unwired: 7 in, 1 out]
                  n260 = Select(t=TRUE, s=w523, f=FALSE) -> (s? t:f=w521:bool)
                }
                n261 = property on="QUIT" class="Bool"(error in=w502, "DisabledEnum"=T19."Disabled and Grayed Out" ("Disabled")) -> ()  [unwired: 1 in, 2 out]
                n262 = flat-sequence {
                  tunnel: w506 -> [_]
                  frame #0 {
                    n263 = local read "VGA"() -> (w517:T2)
                    n264 = Unbundle By Name(w517) -> ("TIME VGA.PULSE WIDTH"=w514:u16, "TIME VGA.FRECUENCY PULSE"=w513:dbl)
                    n265 = property on="vga test" class="Clust (strict)"("Visible"=TRUE) -> ()  [unwired: 2 in, 2 out]
                    n266 = property on="VGA" class="Clust (strict)"("Visible"=FALSE) -> ()  [unwired: 2 in, 2 out]
                    n267 = Bundle By Name(cluster=T14 {"FRECUENCY PULSE"=0.0, "PULSE WIDTH"=0, "CODE GAIN TEST"=0} ("Value (Signaling)"), "CODE GAIN TEST"=u8 0, "PULSE WIDTH"=w514, "FRECUENCY PULSE"=w513) -> (w515:T14)
                    n268 = property on="vga test" class="Clust (strict)"("Val(Sgnl)"=w515) -> ()  [unwired: 2 in, 2 out]
                  }
                }
                n269 = call <vilib>:"Clear Errors.vi"("error in (no error)"=w509) -> ("error out"=w504:errorcluster)  [unwired: 5 in, 1 out]
                n270 = call "FT_Search All Select description.vi"("error in (no error)"=w504, "CTA Test#"=w507) -> ("Select Ft"=w508:T24)  [unwired: 7 in, 2 out]
                n271 = Unbundle By Name(w508) -> ("FT_Handle"=w506:u32)
                n272 = local write "FT_Handle"(w506) -> ()
              }
            }
          }
          event "vga test": Value Change {
            w558 = u32 20 ("Espera acceso USB")
            n273 = event-data() -> ()  [unwired: 1 in, 5 out]
            n274 = local read "FT_Handle"() -> (w559:u32)
            n275 = Unbundle By Name("vga test") -> ("PULSE WIDTH"=w555:u16, "FRECUENCY PULSE"=w553:dbl, "CODE GAIN TEST"=w554:u8)
            n276 = call "VGA_pulso.vi"("Espera acceso USB"=w558, "Frecuencia pulso (0.2 a 1 Mhz)"=w553, "Patrón (E000)"=w555, "ftHandle_in"=w559) -> ("error out"=w560:errorcluster, "ftHandle_out"=w561:u32)  [unwired: 6 in]
            n277 = call "VGA_ganancia.vi"("Espera acceso USB"=w558, "error in 2"=w560, "Ganancia"=w554, "ftHandle_in 2"=w561) -> ()  [unwired: 6 in, 2 out]
          }
          event "Elemensts": Value Change {
            n278 = event-data() -> ()  [unwired: 1 in, 5 out]
            n279 = property on="Valores" class="Arr (strict)"() -> ("Value"=w572:T16[])  [unwired: 2 in, 2 out]
            n280 = for {
              tunnel: [w574] -> w569 mode=indexing
              tunnel: w572 -> [w573] mode=indexing
              n281 = Unbundle By Name(w573) -> ("VOLTAGE SUPPLY ASIC"=w574:dbl)
            }
            n282 = Number To Fractional String(number=w569, width (-)=i16 1, precision (6)=i16 2) -> (F-format string=w568:string[])  [unwired: 1 in]
            n283 = property on="Elemensts" class="LstBox (strict)"("Item Names"=w568) -> ("Value"=w567:i32)  [unwired: 2 in, 2 out]
            n284 = Build Array(w567) -> (w566:i32[])
            n285 = property on="Valores" class="Arr (strict)"("Index Values"=w566) -> ()  [unwired: 2 in, 2 out]
            n286 = local write "Cambios"(TRUE ("Cambios")) -> ()
          }
          event "new": Value Change {
            n287 = event-data() -> ()  [unwired: 1 in, 5 out]
            n288 = call "gui.default values test.vi"() -> ("Values default"=w598:T26)  [unwired: 7 in, 4 out]
            n289 = property on="Valores" class="Arr (strict)"() -> ("Value"=w593:T16[])  [unwired: 2 in, 2 out]
            n290 = Index Array(array=w598, index=1) -> (element=w597:T27)
            n291 = Unbundle By Name(w597) -> ("Vsupply asic"=w648:dbl, "Vsupply asic real"=w577:dbl, "Global Reset"=w579:bool, "IBIAS"=w575:bool, "VALUE IBIAS"=w576:u8, "Test Register??"=w587:bool, "Test ADC??"=w647:bool, "Test ADC set.Repeats ADC"=w646:i32, "Test ADC set.Max Desviation"=w645:dbl, "High ADC means"=w642:dbl[], "Low ADC means"=w641:dbl[], "Test MAX/MIN??"=w638:bool, "Limits Max PN Min NP.Max P Lower"=w637:dbl, "Limits Max PN Min NP.Min P Lower"=w636:dbl, "Limits Max PN Min NP.Max N Lower"=w635:dbl, "Limits Max PN Min NP.Min N Lower"=w634:dbl, "Limits Max PN Min NP.Max P Upper"=w602:dbl, "Limits Max PN Min NP.Min P Upper"=w601:dbl, "Limits Max PN Min NP.Max N Upper"=w600:dbl, "Limits Max PN Min NP.Min N Upper"=w599:dbl, "Test rate scan"=w627:bool, "Vin Rate Scan"=w626:i32[], "High rate scan"=w605:dbl[], "Low rate scan"=w606:dbl[], "Test rate scan adders??"=w621:bool, "Vin Rate Adders"=w620:i32[], "High rate scan add"=w603:dbl[], "Low rate scan add"=w604:dbl[], "Test offset analog??"=w615:bool, "Lim Offset Analog.Max Analog"=w614:dbl, "Lim Offset Analog.Min Analog"=w613:dbl, "Test offset digital??"=w612:bool, "Lim offset Dig.Max Dig"=w611:dbl)
            n292 = Build Array(w604, w603) -> (w619:dbl[][])
            n293 = Build Array(w602, w601, w600, w599) -> (w632:dbl[])
            n294 = Build Array(w606, w605) -> (w623:dbl[][])
            n295 = Build Array(w641, w642) -> (w640:dbl[][])
            n296 = Build Array(w637, w636, w635, w634) -> (w633:dbl[])
            n297 = Transpose 2D Array(2D array=w623) -> (transposed array=w608:dbl[][])
            n298 = Transpose 2D Array(2D array=w640) -> (transposed array=w610:dbl[][])
            n299 = Transpose 2D Array(2D array=w619) -> (transposed array=w607:dbl[][])
            n300 = Build Array(w633, w632) -> (w629:dbl[][])
            n301 = Transpose 2D Array(2D array=w629) -> (transposed array=w609:dbl[][])
            n302 = Number To Fractional String(number=w608, width (-)=i16 1, precision (6)=i16 4) -> (F-format string=w622:string[][])  [unwired: 1 in]
            n303 = Number To Fractional String(number=w610, width (-)=i16 1, precision (6)=i16 4) -> (F-format string=w639:string[][])  [unwired: 1 in]
            n304 = Number To Fractional String(number=w607, width (-)=i16 1, precision (6)=i16 4) -> (F-format string=w616:string[][])  [unwired: 1 in]
            n305 = Number To Fractional String(number=w609, width (-)=i16 1, precision (6)=i16 4) -> (F-format string=w628:string[][])  [unwired: 1 in]
            n306 = Index Array(array=w593, index=0) -> (element=w649:T16)
            n307 = Bundle By Name(cluster=w649, "VOLTAGE SUPPLY ASIC"=w648, "V SUPPLY ASIC REAL"=w577, "GLOBAL RESET"=w579, "IBIAS"=w575, "VALUE IBIAS"=w576, "TEST REGISTER"=w587, "TEST ADC"=w647, "SETUP ADC.NUMBER OF REPETITIONS"=w646, "SETUP ADC.MAX DESVIATION ADC"=w645, "LIMITS MEASUREMENT ADC"=w639, "TEST MAX MIN P/N"=w638, "LIMITS MAX PN MIN NP"=w628, "TEST RATE SCAN"=w627, "VIN ASIC"=w626, "LIMITS RATE SCAN"=w622, "TEST RATE SCAN ADDERS"=w621, "VIN ASIC ADD"=w620, "LIMITS RATE SCAN ADDERS"=w616, "TEST OFFSET ANALOG"=w615, "LIMITS OFFSET ANALOG.MAXIMUM"=w614, "LIMITS OFFSET ANALOG.MINIMUM"=w613, "TEST OFFSET DIGITAL"=w612, "LIMITS OFFSET DIGITAL.MAXIMUM"=w611) -> (w592:T16)
            n308 = Build Array (concatenate)(w593, w592) -> (w582:T16[])
            n309 = Array Size(array=w582) -> (size(s)=w589:i32)
            n310 = property on="Valores" class="Arr (strict)"("Value"=w582) -> (error out=w591:errorcluster)  [unwired: 2 in, 1 out]
            n311 = Decrement(x=w589) -> (x-1=w580:i32)
            n312 = property on="Valores" class="Arr (strict)"(error in=w591, "Val(Sgnl)"=w582) -> ()  [unwired: 1 in, 2 out]
            n313 = for {
              tunnel: [w651] -> w581 mode=indexing
              tunnel: w582 -> [w650] mode=indexing
              n314 = Unbundle By Name(w650) -> ("VOLTAGE SUPPLY ASIC"=w651:dbl)
            }
            n315 = Build Array(w580) -> (w588:i32[])
            n316 = Number To Fractional String(number=w581, width (-)=i16 1, precision (6)=i16 2) -> (F-format string=w583:string[])  [unwired: 1 in]
            n317 = property on="Valores" class="Arr (strict)"("Index Values"=w588) -> ()  [unwired: 2 in, 2 out]
            n318 = property on="Elemensts" class="LstBox (strict)"("EditRow"=w580, "Item Names"=w583) -> ()  [unwired: 2 in, 2 out]
            n319 = local write "Cambios"(TRUE ("Cambios")) -> ()
          }
          event "Load config": Value Change {
            n320 = event-data() -> ()  [unwired: 1 in, 5 out]
            n321 = disable-structure shown="Disabled" {
              disable-tunnel: [w670 _] -> _
              frame Disabled {
                n322 = call <vilib>:"Three Button Dialog.vi"("Window Title (\"\")"="Warning, the configuration file has not been saved!!" ("Window Title (\"\")"), "Right Button Text (\"Cancel\")"="Cancel" ("Right Button Text (\"Cancel\")"), "Center Button Text (\"No\")"="Don't Save & Load" ("Center Button Text (\"No\")"), "Left Button Text (\"Yes\")"="Save File & Load" ("Left Button Text (\"Yes\")"), "message"="The configuration of the test is about to leave memory. It's unsaved changes will be lost.. As you wish to proceed???") -> ("Which Button?"=w666:T28)  [unwired: 6 in]
                n323 = case shown="\"Right Button\"" w666 {
                  tunnel: [machine_estate_configs."Save In Config" ("MACHINE") machine_estate_configs."Load File" ("MACHINE") machine_estate_configs."wait" ("MACHINE") machine_estate_configs."wait" ("MACHINE")] -> w670
                  frame "Left Button", Default {
                    n324 = local write item#-1(TRUE ("Load despues")) -> ()
                  }
                  frame "Center Button" {
                  }
                  frame "Right Button" {
                  }
                  frame "Window Close" {
                  }
                }
              }
              frame Enabled {
              }
            }
            n325 = case shown="True" "Load config" {
              tunnel: [machine_estate_configs."wait" ("MACHINE") w658] -> w653
              frame False {
              }
              frame True {
                n326 = local read "Cambios"() -> (w657:bool)
                n327 = case shown="True" w657 {
                  tunnel: [machine_estate_configs."Load File" ("MACHINE") w660] -> w658
                  frame False {
                  }
                  frame True {
                    n328 = call "Display Message to User"() -> ("Don't Save & Load"=w663:bool)  [unwired: 10 in, 1 out]
                    n329 = Select(t=machine_estate_configs."Load File" ("MACHINE"), s=w663, f=machine_estate_configs."wait" ("MACHINE")) -> (s? t:f=w660:T17)
                  }
                }
              }
            }
          }
          event "copy to new": Value Change {
            n330 = event-data() -> ()  [unwired: 1 in, 5 out]
            n331 = property on="Valores" class="Arr (strict)"() -> ("Value"=w683:T16[], "Index Values"=w690:u32[])  [unwired: 2 in, 2 out]
            n332 = Index Array(array=w690, index=0) -> (element=w688:u32)
            n333 = Index Array(array=w683, index=w688) -> (element=w694:T16)
            n334 = Build Array (concatenate)(w683, w694) -> (w678:T16[])
            n335 = property on="Valores" class="Arr (strict)"("Value"=w678) -> (error out=w686:errorcluster)  [unwired: 2 in, 1 out]
            n336 = property on="Valores" class="Arr (strict)"(error in=w686, "Val(Sgnl)"=w678) -> (error out=w693:errorcluster)  [unwired: 1 in, 1 out]
            n337 = Array Size(array=w678) -> (size(s)=w687:i32)
            n338 = for {
              tunnel: [w696] -> w679 mode=indexing
              tunnel: w678 -> [w695] mode=indexing
              n339 = Unbundle By Name(w695) -> ("VOLTAGE SUPPLY ASIC"=w696:dbl)
            }
            n340 = Decrement(x=w687) -> (x-1=w677:i32)
            n341 = Build Array(w677) -> (w692:i32[])
            n342 = property on="Valores" class="Arr (strict)"(error in=w693, "Index Values"=w692) -> ()  [unwired: 1 in, 2 out]
            n343 = Number To Fractional String(number=w679, width (-)=i16 1, precision (6)=i16 2) -> (F-format string=w680:string[])  [unwired: 1 in]
            n344 = property on="Elemensts" class="LstBox (strict)"("EditRow"=w677, "Item Names"=w680) -> ()  [unwired: 2 in, 2 out]
            n345 = local write "Cambios"(TRUE ("Cambios")) -> ()
          }
          event "delete": Value Change {
            n346 = event-data() -> ()  [unwired: 1 in, 5 out]
            n347 = property on="Valores" class="Arr (strict)"() -> ("Value"=w705:T16[])  [unwired: 2 in, 2 out]
            n348 = Array Size(array=w705) -> (size(s)=w704:i32)
            n349 = Decrement(x=w704) -> (x-1=w700:i32)
            n350 = Greater Or Equal?(x=w700, y=0) -> (x >= y?=w702:bool)
            n351 = case shown="True" w702 {
              frame False {
              }
              frame True {
                w708 = u32[] [0] ("Index Values")
                n352 = property on="Valores" class="Arr (strict)"() -> ("Value"=w715:T16[], "Index Values"=w717:u32[])  [unwired: 2 in, 2 out]
                n353 = Index Array(array=w717, index=0) -> (element=w709:u32)
                n354 = Delete From Array(array=w715, length=1, index=w709) -> (array with subset deleted=w710:T16[])  [unwired: 1 out]
                n355 = for {
                  tunnel: w710 -> [w721] mode=indexing
                  tunnel: [w720] -> w712 mode=indexing
                  n356 = Unbundle By Name(w721) -> ("VOLTAGE SUPPLY ASIC"=w720:dbl)
                }
                n357 = property on="Valores" class="Arr (strict)"("Val(Sgnl)"=w710) -> (error out=w718:errorcluster)  [unwired: 2 in, 1 out]
                n358 = Index Array(array=w708, index=0) -> (element=w706:u32)
                n359 = property on="Valores" class="Arr (strict)"(error in=w718, "Index Values"=w708) -> ()  [unwired: 1 in, 2 out]
                n360 = Number To Fractional String(number=w712, width (-)=i16 1, precision (6)=i16 2) -> (F-format string=w711:string[])  [unwired: 1 in]
                n361 = property on="Elemensts" class="LstBox (strict)"("EditRow"=w706, "Item Names"=w711) -> ()  [unwired: 2 in, 2 out]
              }
            }
            n362 = local write "Cambios"(TRUE ("Cambios")) -> ()
          }
          event "VGA": Value Change {
            n363 = event-data() -> ()  [unwired: 1 in, 5 out]
            n364 = First Call?() -> (First Call?: T/F=w722:bool)
            n365 = case shown="False" w722 {
              frame False {
                n366 = local write "Cambios"(TRUE ("Cambios")) -> ()
              }
              frame True {
              }
            }
          }
          event "VISA Rigol DP832", "VISA Generator Key 81160A", "VISA Oscilloscope Tek MDO3104": Value Change {
            n367 = event-data() -> ()  [unwired: 1 in, 5 out]
            n368 = local write "Cambios"(TRUE ("Cambios")) -> ()
          }
          event "CTA Board": Value Change {
            n369 = event-data() -> ()  [unwired: 1 in, 5 out]
            n370 = local write "Cambios"(TRUE ("Cambios")) -> ()
          }
          event "Config Rigol DP832": Value Change {
            n371 = event-data() -> ()  [unwired: 1 in, 5 out]
            n372 = local write "Cambios"(TRUE ("Cambios")) -> ()
          }
          event "Change value Gen": Value Change {
            n373 = event-data() -> ("NewVal"=w736:bool)  [unwired: 1 in, 4 out]
            n374 = case shown="False" w736 {
              tunnel: w735 -> [_ w745]
              frame False {
              }
              frame True {
                n375 = local read "CONFIG GEN temp"() -> (w740:T1[])
                n376 = Unbundle By Name(w745) -> ("Config HW"=w744:T4)
                n377 = call "GUI.Config Pulse generator.vi"("Config HW"=w744, "CONFIG GEN origen"=w740) -> ("error out"=w742:errorcluster, "Array pulse Out"=w739:T1[])  [unwired: 8 in]
                n378 = for {
                  tunnel: w739 -> [w759] mode=indexing
                  tunnel: [w746] -> w743 mode=indexing
                  n379 = Unbundle By Name(w759) -> ("Amplitude"=w757:dbl, "Frequency"=w751:dbl, "Width Time"=w752:dbl, "Load"=w753:dbl)
                  n380 = Format Value(format string="%#_6pHz", value (0)=w751) -> (output string=w749:string)  [unwired: 1 in]
                  n381 = Format Value(format string="%#_6pV", value (0)=w757) -> (output string=w750:string)  [unwired: 1 in]
                  n382 = Format Value(format string="%#_6ps", value (0)=w752) -> (output string=w748:string)  [unwired: 1 in]
                  n383 = Format Value(format string="%#_6pW", value (0)=w753) -> (output string=w747:string)  [unwired: 1 in]
                  n384 = Build Array(w750, w749, w748, w747) -> (w746:string[])
                }
                "Values Gen" <- w743
                n385 = call <vilib>:"Clear Errors.vi"("error in (no error)"=w742) -> ()  [unwired: 5 in, 2 out]
                n386 = local write "Cambios"(TRUE ("f")) -> ()
                n387 = local write "CONFIG GEN temp"(w739) -> ()
              }
            }
          }
          event "QUIT": Value Change {
            n388 = event-data() -> ()  [unwired: 1 in, 5 out]
            n389 = local read "Cambios"() -> (w760:bool)
            n390 = case shown="True" w760 {
              tunnel: [TRUE w774] -> w762
              tunnel: [machine_estate_configs."quit" ("MACHINE") w773] -> w761
              frame False {
              }
              frame True {
                n391 = call <vilib>:"Three Button Dialog.vi"("Keyboard Shortcuts (Left is <Enter>)"=T20 {"Left Button Key Shortcut"={"Control"=FALSE, "Shift"=TRUE, "Key"="S"}, "Center Button Key Shortcut"={"Control"=FALSE, "Shift"=TRUE, "Key"="Q"}, "Right Button Key Shortcut"={"Control"=TRUE, "Shift"=FALSE, "Key"="C"}}, "Window Title (\"\")"="Warning, the configuration file has not been saved!!" ("Window Title (\"\")"), "Right Button Text (\"Cancel\")"="Cancel" ("Right Button Text (\"Cancel\")"), "Center Button Text (\"No\")"="Don't Save & Quit" ("Center Button Text (\"No\")"), "Left Button Text (\"Yes\")"="Save File" ("Left Button Text (\"Yes\")"), "message"="The configuration of the test is about to leave memory.\nIt's unsaved changes will be lost..\nAs you wish to proceed???") -> ("Which Button?"=w769:T28)  [unwired: 5 in]
                n392 = case shown="\"Left Button\", Default" w769 {
                  tunnel: [FALSE TRUE FALSE FALSE] -> w774
                  tunnel: [machine_estate_configs."Save In Config" ("MACHINE") machine_estate_configs."quit" ("MACHINE") machine_estate_configs."wait" ("MACHINE") machine_estate_configs."wait" ("MACHINE")] -> w773
                  frame "Left Button", Default {
                  }
                  frame "Center Button" {
                  }
                  frame "Right Button" {
                  }
                  frame "Window Close" {
                  }
                }
              }
            }
          }
          event "save config": Value Change {
            n393 = event-data() -> ()  [unwired: 1 in, 5 out]
          }
        }
      }
      frame "Valores>Test" {
        n394 = Unbundle By Name(w799) -> ("Config Test"=w800:T6)
        n395 = local read "Valores"() -> (w795:T16[])
        n396 = Index Array(array=w800, index=0) -> (element=w802:T7)
        n397 = local read "VISA Oscilloscope Tek MDO3104"() -> (w788:refnum<visa-resource-name>)
        n398 = property on="VALUES VGA" class="Tbl (strict)"() -> ("Row Headers[]"=w791:string[])  [unwired: 2 in, 2 out]
        n399 = local read "VISA Generator Key 81160A"() -> (w789:refnum<visa-resource-name>)
        n400 = local read "VGA"() -> (w794:T2)
        n401 = for {
          tunnel: w795 -> [w870] mode=indexing
          tunnel: w802 -> [w869]
          tunnel: [w852] -> w787 mode=indexing
          n402 = Unbundle By Name(w870) -> ("VOLTAGE SUPPLY ASIC"=w868:dbl, "V SUPPLY ASIC REAL"=w817:dbl, "GLOBAL RESET"=w818:bool, "IBIAS"=w816:bool, "VALUE IBIAS"=w815:u8, "TEST REGISTER"=w825:bool, "TEST ADC"=w867:bool, "SETUP ADC.NUMBER OF REPETITIONS"=w866:i32, "SETUP ADC.MAX DESVIATION ADC"=w865:dbl, "LIMITS MEASUREMENT ADC"=w856:string[][], "TEST MAX MIN P/N"=w864:bool, "LIMITS MAX PN MIN NP"=w851:string[][], "TEST RATE SCAN"=w863:bool, "VIN ASIC"=w862:i32[], "LIMITS RATE SCAN"=w846:string[][], "TEST RATE SCAN ADDERS"=w861:bool, "VIN ASIC ADD"=w860:i32[], "LIMITS RATE SCAN ADDERS"=w821:string[][], "TEST OFFSET ANALOG"=w859:bool, "LIMITS OFFSET ANALOG.MAXIMUM"=w842:dbl, "LIMITS OFFSET ANALOG.MINIMUM"=w841:dbl, "TEST OFFSET DIGITAL"=w858:bool, "LIMITS OFFSET DIGITAL.MAXIMUM"=w857:dbl)
          n403 = Fract/Exp String To Number(string=w821) -> (number=w822:dbl[][])  [unwired: 3 in, 1 out]
          n404 = Fract/Exp String To Number(string=w846) -> (number=w845:dbl[][])  [unwired: 3 in, 1 out]
          n405 = Fract/Exp String To Number(string=w851) -> (number=w828:dbl[][])  [unwired: 3 in, 1 out]
          n406 = Index Array(array=w845, index (col) #1=1 ("index (row)"), index (col) #2=0 ("index (row)")) -> (element #1=w844:dbl[], element #2=w843:dbl[])  [unwired: 2 in]
          n407 = Fract/Exp String To Number(string=w856) -> (number=w855:dbl[][])  [unwired: 3 in, 1 out]
          n408 = Index Array(array=w822, index (col) #1=1 ("index (row)"), index (col) #2=0 ("index (row)")) -> (element #1=w820:dbl[], element #2=w819:dbl[])  [unwired: 2 in]
          n409 = Index Array(array=w828, index (col) #1=0 ("index (row)"), index (col) #2=1 ("index (row)")) -> (element #1=w850:dbl[], element #2=w848:dbl[])  [unwired: 2 in]
          n410 = Index Array(array=w855, index (col) #1=0 ("index (row)"), index (col) #2=1 ("index (row)")) -> (element #1=w854:dbl[], element #2=w853:dbl[])  [unwired: 2 in]
          n411 = Index Array(array=w850, index #1=0 ("index")) -> (element #1=w838:dbl, element #2=w837:dbl, element #3=w836:dbl, element #4=w835:dbl)  [unwired: 3 in]
          n412 = Index Array(array=w848, index #1=0 ("index")) -> (element #1=w834:dbl, element #2=w833:dbl, element #3=w832:dbl, element #4=w831:dbl)  [unwired: 3 in]
          n413 = Bundle By Name(cluster=w869, "Vasic"=w868, "Vasic real f.a."=w817, "Global Reset"=w818, "IBIAS"=w816, "VALUE IBIAS"=w815, "Test Register?"=w825, "Test ADC?"=w867, "Test ADC.Repeats ADC"=w866, "Test ADC.Max Desviation"=w865, "Limits ADC.Low"=w854, "Limits ADC.High"=w853, "Test Max PN Min NP?"=w864, "Limits Max PN Min NP.Max P Lower"=w838, "Limits Max PN Min NP.Min P Lower"=w837, "Limits Max PN Min NP.Max N Lower"=w836, "Limits Max PN Min NP.Min N Lower"=w835, "Limits Max PN Min NP.Max P Upper"=w834, "Limits Max PN Min NP.Min P Upper"=w833, "Limits Max PN Min NP.Max N Upper"=w832, "Limits Max PN Min NP.Min N Upper"=w831, "Test Rate Scan?"=w863, "Vin Rate Scan"=w862, "Limits Rate Scan.High"=w844, "Limits Rate Scan.Low"=w843, "Test Rate Scan Adders?"=w861, "Vin Rate Adders"=w860, "Limits Rate Scan adders.High"=w820, "Limits Rate Scan adders.Low"=w819, "Test offset analog?"=w859, "Lim Offset Analog.Max Analog"=w842, "Lim Offset Analog.Min Analog"=w841, "Test offset digital?"=w858, "Lim offset Dig.Max Dig"=w857) -> (w852:T7)
        }
        n414 = local read "Config Rigol DP832"() -> (w793:T15)
        n415 = local read "VISA Rigol DP832"() -> (w792:refnum<visa-resource-name>)
        n416 = local read "CTA Board"() -> (w790:string)
        n417 = Unbundle By Name(w794) -> ("VALUES VGA"=w807:string[][], "TIME VGA.PULSE WIDTH"=w806:u16, "TIME VGA.FRECUENCY PULSE"=w805:dbl)
        n418 = local read "CONFIG GEN temp"() -> (w786:T1[])
        n419 = Fract/Exp String To Number(string=w791) -> (number=w813:dbl[])  [unwired: 3 in, 1 out]
        n420 = Divide(x=w813, y=1000.0) -> (x/y=w812:dbl[])
        n421 = Index Array(array=w807, index (col) #1=1 ("disabled index (col)"), index (col) #2=0 ("index (col)")) -> (element #1=w810:string[], element #2=w808:string[])  [unwired: 2 in]
        n422 = Fract/Exp String To Number(string=w810) -> (number=w811:dbl[])  [unwired: 3 in, 1 out]
        n423 = Decimal String To Number(string=w808) -> (number=w809:i32[])  [unwired: 2 in, 1 out]
        n424 = Bundle By Name(cluster=w799, "Config HW.Config Rigol DP832"=w793, "Config HW.VISA Key 81160A"=w789, "Config HW.VISA Tek MDO3104"=w788, "Config HW.VISA Rigol DP832"=w792, "Config HW.CTA Test#"=w790, "Config VGA.Theoretical Voltage"=w812, "Config VGA.Real Voltage"=w811, "Config VGA.VGA Gain"=w809, "Config VGA.Pulse Width"=w806, "Config VGA.Frecuency Pulse"=w805, "CONFIG GEN"=w786, "Config Test"=w787) -> (w798:T18)
      }
      frame "Save In Config" {
        n425 = Unbundle By Name(w877) -> ("Config Test"=w899:T6)
        n426 = Index Array(array=w899, index=0) -> (element=w897:T7)
        n427 = local read "VGA"() -> (w874:T2)
        n428 = for {
          tunnel: "Valores" -> [w955] mode=indexing
          tunnel: w897 -> [w954]
          tunnel: [w938] -> w882 mode=indexing
          n429 = Unbundle By Name(w955) -> ("VOLTAGE SUPPLY ASIC"=w953:dbl, "V SUPPLY ASIC REAL"=w902:dbl, "GLOBAL RESET"=w903:bool, "IBIAS"=w901:bool, "VALUE IBIAS"=w900:u8, "TEST REGISTER"=w911:bool, "TEST ADC"=w952:bool, "SETUP ADC.NUMBER OF REPETITIONS"=w951:i32, "SETUP ADC.MAX DESVIATION ADC"=w950:dbl, "LIMITS MEASUREMENT ADC"=w942:string[][], "TEST MAX MIN P/N"=w949:bool, "LIMITS MAX PN MIN NP"=w937:string[][], "TEST RATE SCAN"=w948:bool, "VIN ASIC"=w947:i32[], "LIMITS RATE SCAN"=w932:string[][], "TEST RATE SCAN ADDERS"=w946:bool, "VIN ASIC ADD"=w945:i32[], "LIMITS RATE SCAN ADDERS"=w906:string[][], "TEST OFFSET ANALOG"=w910:bool, "LIMITS OFFSET ANALOG.MAXIMUM"=w928:dbl, "LIMITS OFFSET ANALOG.MINIMUM"=w927:dbl, "TEST OFFSET DIGITAL"=w944:bool, "LIMITS OFFSET DIGITAL.MAXIMUM"=w943:dbl)
          n430 = Fract/Exp String To Number(string=w937) -> (number=w914:dbl[][])  [unwired: 3 in, 1 out]
          n431 = Fract/Exp String To Number(string=w906) -> (number=w907:dbl[][])  [unwired: 3 in, 1 out]
          n432 = Fract/Exp String To Number(string=w942) -> (number=w941:dbl[][])  [unwired: 3 in, 1 out]
          n433 = Fract/Exp String To Number(string=w932) -> (number=w931:dbl[][])  [unwired: 3 in, 1 out]
          n434 = Index Array(array=w914, index (col) #1=0 ("index (row)"), index (col) #2=1 ("index (row)")) -> (element #1=w936:dbl[], element #2=w934:dbl[])  [unwired: 2 in]
          n435 = Index Array(array=w907, index (col) #1=1 ("index (row)"), index (col) #2=0 ("index (row)")) -> (element #1=w905:dbl[], element #2=w904:dbl[])  [unwired: 2 in]
          n436 = Index Array(array=w941, index (col) #1=0 ("index (row)"), index (col) #2=1 ("index (row)")) -> (element #1=w940:dbl[], element #2=w939:dbl[])  [unwired: 2 in]
          n437 = Index Array(array=w936, index #1=0 ("index")) -> (element #1=w924:dbl, element #2=w923:dbl, element #3=w922:dbl, element #4=w921:dbl)  [unwired: 3 in]
          n438 = Index Array(array=w934, index #1=0 ("index")) -> (element #1=w920:dbl, element #2=w919:dbl, element #3=w918:dbl, element #4=w917:dbl)  [unwired: 3 in]
          n439 = Index Array(array=w931, index (col) #1=1 ("index (row)"), index (col) #2=0 ("index (row)")) -> (element #1=w930:dbl[], element #2=w929:dbl[])  [unwired: 2 in]
          n440 = Bundle By Name(cluster=w954, "Vasic"=w953, "Vasic real f.a."=w902, "Global Reset"=w903, "IBIAS"=w901, "VALUE IBIAS"=w900, "Test Register?"=w911, "Test ADC?"=w952, "Test ADC.Repeats ADC"=w951, "Test ADC.Max Desviation"=w950, "Limits ADC.Low"=w940, "Limits ADC.High"=w939, "Test Max PN Min NP?"=w949, "Limits Max PN Min NP.Max P Lower"=w924, "Limits Max PN Min NP.Min P Lower"=w923, "Limits Max PN Min NP.Max N Lower"=w922, "Limits Max PN Min NP.Min N Lower"=w921, "Limits Max PN Min NP.Max P Upper"=w920, "Limits Max PN Min NP.Min P Upper"=w919, "Limits Max PN Min NP.Max N Upper"=w918, "Limits Max PN Min NP.Min N Upper"=w917, "Test Rate Scan?"=w948, "Vin Rate Scan"=w947, "Limits Rate Scan.High"=w930, "Limits Rate Scan.Low"=w929, "Test Rate Scan Adders?"=w946, "Vin Rate Adders"=w945, "Limits Rate Scan adders.High"=w905, "Limits Rate Scan adders.Low"=w904, "Test offset analog?"=w910, "Lim Offset Analog.Max Analog"=w928, "Lim Offset Analog.Min Analog"=w927, "Test offset digital?"=w944, "Lim offset Dig.Max Dig"=w943) -> (w938:T7)
        }
        n441 = property on="CTA Board" class="CmbBox"() -> ("Value"=w881:string)  [unwired: 2 in, 2 out]
        n442 = Unbundle By Name(w874) -> ("VALUES VGA"=w892:string[][], "TIME VGA.PULSE WIDTH"=w893:u16, "TIME VGA.FRECUENCY PULSE"=w894:dbl)
        n443 = local read "VISA Oscilloscope Tek MDO3104"() -> (w872:refnum<visa-resource-name>)
        n444 = local read "VISA Generator Key 81160A"() -> (w873:refnum<visa-resource-name>)
        n445 = property on="VALUES VGA" class="Tbl (strict)"() -> ("Row Headers[]"=w887:string[])  [unwired: 2 in, 2 out]
        n446 = local read "Config Rigol DP832"() -> (w875:T15)
        n447 = local read "VISA Rigol DP832"() -> (w876:refnum<visa-resource-name>)
        n448 = Fract/Exp String To Number(string=w887) -> (number=w884:dbl[])  [unwired: 3 in, 1 out]
        n449 = local read "CONFIG GEN temp"() -> (w871:T1[])
        n450 = Divide(x=w884, y=1000.0) -> (x/y=w885:dbl[])
        n451 = Index Array(array=w892, index (col) #1=1 ("disabled index (col)"), index (col) #2=0 ("index (col)")) -> (element #1=w889:string[], element #2=w891:string[])  [unwired: 2 in]
        n452 = Fract/Exp String To Number(string=w889) -> (number=w888:dbl[])  [unwired: 3 in, 1 out]
        n453 = Decimal String To Number(string=w891) -> (number=w890:i32[])  [unwired: 2 in, 1 out]
        n454 = Bundle By Name(cluster=w877, "Config HW.Config Rigol DP832"=w875, "Config HW.VISA Key 81160A"=w873, "Config HW.VISA Tek MDO3104"=w872, "Config HW.VISA Rigol DP832"=w876, "Config HW.CTA Test#"=w881, "Config VGA.Theoretical Voltage"=w885, "Config VGA.Real Voltage"=w888, "Config VGA.VGA Gain"=w890, "Config VGA.Pulse Width"=w893, "Config VGA.Frecuency Pulse"=w894, "CONFIG GEN"=w871, "Config Test"=w882) -> (w879:T18)
      }
      frame "Default values" {
        w966 = 0 ("Elemensts")
        n455 = call "gui.default values test.vi"() -> ("Config Rigol DP832"=w970:T15, "Config Hw"=w985:T29, "Config VGA"=w986:T11, "Values default"=w987:T26, "Values Generator"=w956:T1[])  [unwired: 7 in]
        n456 = local read "Valores"() -> (w988:T16[])
        n457 = Unbundle By Name(w985) -> ("VISA Rigol DP832"=w971:refnum<visa-resource-name>, "VISA Tek MDO3104"=w961:refnum<visa-resource-name>, "VISA Key 81160a"=w960:refnum<visa-resource-name>, "CTA Test#"=w967:string)
        n458 = for {
          tunnel: w988 -> [w1067]
          tunnel: w987 -> [w1065] mode=indexing
          shift-right: [w1016] -> w972
          shift-left: T16[] [] -> [w1014]
          tunnel: [w1006] -> w962 mode=indexing
          n459 = Unbundle By Name(w1065) -> ("Vsupply asic"=w1007:dbl, "Vsupply asic real"=w1005:dbl, "Global Reset"=w1010:bool, "IBIAS"=w1004:bool, "VALUE IBIAS"=w1003:u8, "Test Register??"=w1013:bool, "Test ADC??"=w1064:bool, "Test ADC set.Repeats ADC"=w1063:i32, "Test ADC set.Max Desviation"=w1062:dbl, "High ADC means"=w1059:dbl[], "Low ADC means"=w1058:dbl[], "Test MAX/MIN??"=w1055:bool, "Limits Max PN Min NP.Max P Lower"=w1054:dbl, "Limits Max PN Min NP.Min P Lower"=w1053:dbl, "Limits Max PN Min NP.Max N Lower"=w1052:dbl, "Limits Max PN Min NP.Min N Lower"=w1051:dbl, "Limits Max PN Min NP.Max P Upper"=w1021:dbl, "Limits Max PN Min NP.Min P Upper"=w1020:dbl, "Limits Max PN Min NP.Max N Upper"=w1019:dbl, "Limits Max PN Min NP.Min N Upper"=w1018:dbl, "Test rate scan"=w1045:bool, "Vin Rate Scan"=w1044:i32[], "High rate scan"=w1024:dbl[], "Low rate scan"=w1025:dbl[], "Test rate scan adders??"=w1039:bool, "Vin Rate Adders"=w1038:i32[], "High rate scan add"=w1022:dbl[], "Low rate scan add"=w1023:dbl[], "Test offset analog??"=w1033:bool, "Lim Offset Analog.Max Analog"=w1032:dbl, "Lim Offset Analog.Min Analog"=w1031:dbl, "Test offset digital??"=w1030:bool, "Lim offset Dig.Max Dig"=w1029:dbl)
          n460 = Build Array(w1058, w1059) -> (w1057:dbl[][])
          n461 = Build Array(w1054, w1053, w1052, w1051) -> (w1050:dbl[])
          n462 = Build Array(w1021, w1020, w1019, w1018) -> (w1049:dbl[])
          n463 = Build Array(w1025, w1024) -> (w1041:dbl[][])
          n464 = Build Array(w1023, w1022) -> (w1037:dbl[][])
          n465 = Transpose 2D Array(2D array=w1057) -> (transposed array=w1028:dbl[][])
          n466 = Transpose 2D Array(2D array=w1041) -> (transposed array=w1027:dbl[][])
          n467 = Build Array(w1050, w1049) -> (w1012:dbl[][])
          n468 = Transpose 2D Array(2D array=w1037) -> (transposed array=w1026:dbl[][])
          n469 = Transpose 2D Array(2D array=w1012) -> (transposed array=w1011:dbl[][])
          n470 = Number To Fractional String(number=w1028, width (-)=i16 1, precision (6)=i16 4) -> (F-format string=w1056:string[][])  [unwired: 1 in]
          n471 = Number To Fractional String(number=w1027, width (-)=i16 1, precision (6)=i16 4) -> (F-format string=w1040:string[][])  [unwired: 1 in]
          n472 = Number To Fractional String(number=w1026, width (-)=i16 1, precision (6)=i16 4) -> (F-format string=w1034:string[][])  [unwired: 1 in]
          n473 = Number To Fractional String(number=w1011, width (-)=i16 1, precision (6)=i16 4) -> (F-format string=w1046:string[][])  [unwired: 1 in]
          n474 = Index Array(array=w1067, index=0) -> (element=w1066:T16)
          n475 = Bundle By Name(cluster=w1066, "VOLTAGE SUPPLY ASIC"=w1007, "V SUPPLY ASIC REAL"=w1005, "GLOBAL RESET"=w1010, "IBIAS"=w1004, "VALUE IBIAS"=w1003, "TEST REGISTER"=w1013, "TEST ADC"=w1064, "SETUP ADC.NUMBER OF REPETITIONS"=w1063, "SETUP ADC.MAX DESVIATION ADC"=w1062, "LIMITS MEASUREMENT ADC"=w1056, "TEST MAX MIN P/N"=w1055, "LIMITS MAX PN MIN NP"=w1046, "TEST RATE SCAN"=w1045, "VIN ASIC"=w1044, "LIMITS RATE SCAN"=w1040, "TEST RATE SCAN ADDERS"=w1039, "VIN ASIC ADD"=w1038, "LIMITS RATE SCAN ADDERS"=w1034, "TEST OFFSET ANALOG"=w1033, "LIMITS OFFSET ANALOG.MAXIMUM"=w1032, "LIMITS OFFSET ANALOG.MINIMUM"=w1031, "TEST OFFSET DIGITAL"=w1030, "LIMITS OFFSET DIGITAL.MAXIMUM"=w1029) -> (w1015:T16)
          n476 = Build Array (concatenate)(w1014, w1015) -> (w1016:T16[])
          n477 = Number To Fractional String(number=w1007, width (-)=i16 1, precision (6)=i16 2) -> (F-format string=w1006:string)  [unwired: 1 in]
        }
        n478 = Unbundle By Name(w986) -> ("Real Voltage"=w979:dbl[], "VGA Gain"=w977:u8[], "Pulse Width"=w981:u16, "Frecuency Pulse"=w982:dbl)
        n479 = local write "CONFIG GEN temp"(w956) -> ()
        n480 = for {
          tunnel: w956 -> [w1002] mode=indexing
          tunnel: [w989] -> w959 mode=indexing
          n481 = Unbundle By Name(w1002) -> ("Amplitude"=w1000:dbl, "Frequency"=w994:dbl, "Width Time"=w995:dbl, "Load"=w996:dbl)
          n482 = Format Value(format string="%#_6pHz", value (0)=w994) -> (output string=w992:string)  [unwired: 1 in]
          n483 = Format Value(format string="%#_6pV", value (0)=w1000) -> (output string=w993:string)  [unwired: 1 in]
          n484 = Format Value(format string="%#_6ps", value (0)=w995) -> (output string=w991:string)  [unwired: 1 in]
          n485 = Format Value(format string="%#_6pOhm", value (0)=w996) -> (output string=w990:string)  [unwired: 1 in]
          n486 = Build Array(w993, w992, w991, w990) -> (w989:string[])
        }
        n487 = Number To Fractional String(number=w979, width (-)=i16 1, precision (6)=i16 4) -> (F-format string=w973:string[])  [unwired: 1 in]
        n488 = Number To Decimal String(number=w977) -> (decimal integer string=w974:string[])  [unwired: 1 in]
        n489 = Build Array(w974, w973) -> (w976:string[][])
        n490 = Transpose 2D Array(2D array=w976) -> (transposed array=w975:string[][])
        n491 = property on="CTA Board" class="CmbBox"("Value"=w967) -> ()  [unwired: 2 in, 2 out]
        n492 = Bundle("CTA Test#"=w967, "CTA Test#"=w967) -> (w969:cluster{"CTA Test#":string, "CTA Test#":string})  [unwired: 1 in]
        n493 = Build Array(w969) -> (w968:T21)
        n494 = property on="Values Gen" class="Tbl (strict)"("Value"=w959) -> ()  [unwired: 2 in, 2 out]
        n495 = local write "VISA Oscilloscope Tek MDO3104"(w961) -> ()
        n496 = local write "VISA Generator Key 81160A"(w960) -> ()
        n497 = local write "Config Rigol DP832"(w970) -> ()
        n498 = local write "VISA Rigol DP832"(w971) -> ()
        n499 = property on="CTA Board" class="CmbBox"("Strings And Values[]"=w968) -> ()  [unwired: 2 in, 2 out]
        n500 = local read "VGA"() -> (w984:T2)
        n501 = Bundle By Name(cluster=w984, "VALUES VGA"=w975, "TIME VGA.PULSE WIDTH"=w981, "TIME VGA.FRECUENCY PULSE"=w982) -> (w983:T2)
        n502 = property on="VGA" class="Clust (strict)"("Value"=w983) -> ()  [unwired: 2 in, 2 out]
        n503 = property on="Elemensts" class="LstBox (strict)"("Value"=w966, "EditRow"=w966, "Item Names"=w962) -> ()  [unwired: 2 in, 2 out]
        n504 = property on="Valores" class="Arr (strict)"("Value"=w972) -> ()  [unwired: 2 in, 2 out]
        n505 = local write "Cambios"(TRUE ("Cambios")) -> ()
      }
    }
  }
  n506 = flat-sequence {
    tunnel: w8 -> [_]
    tunnel: [w1068] -> w2
    frame #0 {
      n507 = local read "Path Config file"() -> (w1068:path)
      "Path out" <- w1068
    }
  }
  n508 = disable-structure shown="Disabled" {
    disable-tunnel: w2 -> [w1069 _]
    frame Disabled {
      n509 = flat-sequence {
        tunnel: w1069 -> [_]
        frame #0 {
          n510 = control-ref of="This VI"() -> (w1070:refnum<vi>)
          n511 = invoke class="VI" method="FP.Close"(reference=w1070) -> ()  [unwired: 2 in, 3 out]
        }
      }
    }
    frame Enabled {
    }
  }
